vi "MultiPAS-IV.vi"() -> ()   [LabVIEW 2011]
uses:
  <vilib>/Analysis/4window.llb/windowTd.ctl
  sub/QMH/QMH Add Message to Queue (Single Element).vi
  sub/QMH/QMH Add Message to Queue (Array).vi
  sub/laserDiagnose_IV.vi
  <vilib>/Instr/_visa.llb/VISA Configure Serial Port (Instr).vi
  sub/lasersSetFrequencies_IV.vi
  sub/absCalcPlot_IV.vi
  <vilib>/measure/maspectr.llb/FFT Spectrum (Mag-Phase) for 1 Chan.vi
  sub/fftGetMags_IV.vi
  sub/rollingAverage_IV.vi
  sub/micUnbundle_IV.vi
  sub/pdNormalize_IV.vi
  <vilib>/measure/NI_MAPro.lvlib
  <vilib>/Analysis/NI_AALPro.lvlib
panel:
  in  "785 Emission":bool
  in  "785 Power (mW)":dbl(slide)=100.0 min=0.0 max=100.0 step=1.0 scale=0.0..100.0
  out "PAS Save":bool caption="Overtemp"
  in  "Data 2":i32[][](array[numeric])=[[-16374, -7248, 2543, 12030, 20279, 26487, 30037, 30583, 28073, 22744, 15131, 5976, -3818, -13288, -21504, -27663, -31155, -31636, -29064, -23686, -16036, -6862, 2936, 12388, 20571, 26684, 30122, 30546, 27911, 22483, 14793, 5595, -4207, -13644, -21795, -27855, -31232, -31591, -28898, -23423, -15695, -6476, 3323, 12743, 20858, 26873, 30194, 30492, 27744, 22213, 14447, 5207, -4597, -14002, -22082, -28044, -31304, -31540, -28731, -23149, -15348, -6093, 3713, 13101, 21145, 27063, 30265, 30442, 27576, 21943, 14103, 4822, -4984, -14354, -22365, -28230, -31373, -31485, -28556, -22876, -14998, -5702, 4104, 13452, 21428, 27245, 30335, 30388, 27400, 21669, 13754, 4435, -5375, -14705, -22643, -28407, -31436, -31426, -28378, -22598, -14648, -5314, 4497, 13803, 21706, 27423, 30394, 30325, 27221, 21390, 13402, 4045, -5763, -15056, -22921, -28586, -31496, -31361, -28198, -22319, -14297, -4924, 4879, 14151, 21982, 27597, 30451, 30257, 27038, 21107, 13050, 3658, -6149, -15402, -23193, -28754, -31546, -31290, -28010, -22033, -13944, -4536, 5266, 14498, 22252, 27767, 30500, 30184, 26849, 20821, 12696, 3267, -6535, -15748, -23462, -28924, -31596, -31216, -27821, -21748, -13587, -4147, 5653, 14838, 22519, 27930, 30549, 30110, 26658, 20535, 12337, 2878, -6919, -16089, -23727, -29087, -31641, -31137, -27627, -21457, -13229, -3753, 6038, 15181, 22786, 28093, 30591, 30031, 26461, 20243, 11979, 2485, -7303, -16428, -23991, -29244, -31678, -31053, -27426, -21159, -12867, -3360, 6424, 15524, 23043, 28252, 30633, 29946, 26262, 19946, 11617, 2096, -7686, -16764, -24246, -29398, -31712, -30964, -27224, -20862, -12503, -2971, 6803, 15859, 23301, 28401, 30661, 29852, 26058, 19648, 11254, 1703, -8069, -17099, -24500, -29547, -31741, -30870, -27018, -20562, -12138, -2575, 7188, 16192, 23556, 28549, 30689, 29756, 25848, 19348, 10891, 1312, -8448, -17430, -24753, -29691, -31765, -30773, -26806, -20259, -11775, -2186, 7566, 16521, 23801, 28690, 30709, 29656, 25634, 19038, 10523, 919, -8831, -17762, -24997, -29833, -31788, -30672, -26593, -19955, -11409, -1792, 7944, 16850, 24047, 28830, 30724, 29548, 25416, 18729, 10152, 523, -9212, -18092, -25245, -29969, -31805, -30566, -26375, -19647, -11041, -1403, 8319, 17173, 24287, 28963, 30734, 29436, 25192, 18418, 9781, 130, -9587, -18413, -25481, -30101, -31814, -30449, -26150, -19332, -10666, -1007, 8697, 17497, 24524, 29090, 30745, 29325, 24968, 18105, 9408, -263, -9962, -18735, -25718, -30228, -31820, -30334, -25921, -19016, -10296, -618, 9072, 17814, 24756, 29213, 30746, 29202, 24738, 17787, 9036, -657, -10338, -19058, -25951, -30350, -31818, -30214, -25690, -18699, -9922, -224, 9442, 18128, 24984, 29330, 30738, 29078, 24502, 17466, 8658, -1050, -10710, -19371, -26178, -30467, -31814, -30088, -25458, -18382, -9550, 167, 9812, 18440, 25206, 29443, 30732, 28947, 24264, 17143, 8281, -1445, -11083, -19685, -26404, -30581, -31807, -29959, -25221, -18059, -9175, 556, 10178, 18750, 25426, 29548, 30718, 28809, 24018, 16812, 7901, -1842, -11457, -19996, -26624, -30690, -31795, -29824, -24980, -17733, -8799, 950, 10549, 19058, 25643, 29655, 30700, 28673, 23773, 16484, 7523, -2235, -11824, -20304, -26840, -30793, -31772, -29682, -24731, -17402, -8415, 1341, 10916, 19363, 25856, 29755, 30677, 28528, 23522, 16151, 7141, -2626, -12191, -20607, -27051, -30891, -31746, -29536, -24481, -17070, -8035, 1733, 11280, 19664, 26064, 29851, 30648, 28381, 23272, 15818, 6762, -3019, -12555, -20906, -27258, -30984, -31717, -29391, -24226, -16736, -7655, 2128, 11641, 19962, 26270, 29940, 30615, 28229, 23013, 15483, 6376, -3409, -12914, -21204, -27459, -31071, -31684, -29236, -23967, -16398, -7271, 2515, 12005, 20258, 26468, 30024, 30577, 28072, 22753, 15143, 5990, -3802, -13276, -21497, -27660, -31157, -31643, -29076, -23707, -16058, -6886, 2908, 12363, 20550, 26666, 30107, 30536, 27914, 22489, 14805, 5607, -4192, -13633, -21787, -27849, -31230, -31597, -28911, -23438, -15716, -6501, 3298, 12719, 20839, 26858, 30182, 30488, 27744, 22223, 14459, 5225, -4579, -13988, -22071, -28040, -31304, -31549, -28743, -23167, -15368, -6113, 3693, 13076, 21126, 27047, 30255, 30438, 27576, 21950, 14113, 4837, -4971, -14340, -22354, -28224, -31375, -31494, -28570, -22895, -15022, -5725, 4080, 13430, 21408, 27230, 30324, 30384, 27402, 21676, 13766, 4449, -5360, -14694, -22636, -28409, -31440, -31436, -28397, -22617, -14674, -5338, 4467, 13781, 21686, 27408, 30385, 30320, 27224, 21398, 13418, 4062, -5748, -15044, -22913, -28584, -31498, -31368, -28212, -22339, -14321, -4948, 4856, 14131, 21963, 27583, 30440, 30254, 27042, 21118, 13062, 3669, -6137, -15390, -23183, -28751, -31551, -31297, -28024, -22049, -13962, -4556, 5245, 14476, 22235, 27754, 30497, 30186, 26857, 20834, 12710, 3283, -6519, -15733, -23453, -28921, -31600, -31226, -27837, -21765, -13610, -4168, 5628, 14820, 22502, 27918, 30540, 30109, 26664, 20544, 12354, 2891, -6906, -16074, -23719, -29085, -31646, -31148, -27642, -21475, -13251, -3777, 6014, 15160, 22765, 28078, 30583, 30027, 26468, 20251, 11994, 2501, -7292, -16415, -23980, -29242, -31682, -31064, -27443, -21181, -12892, -3386, 6397, 15501, 23026, 28238, 30624, 29944, 26269, 19959, 11633, 2110, -7673, -16753, -24239, -29395, -31719, -30974, -27239, -20882, -12528, -2993, 6782, 15835, 23285, 28390, 30651, 29852, 26063, 19660, 11271, 1720, -8053, -17087, -24493, -29546, -31746, -30880, -27031, -20583, -12163, -2599, 7166, 16173, 23538, 28538, 30684, 29758, 25853, 19356, 10906, 1327, -8433, -17416, -24743, -29688, -31769, -30782, -26821, -20280, -11797, -2208, 7543, 16501, 23786, 28680, 30704, 29656, 25642, 19053, 10540, 936, -8814, -17747, -24989, -29827, -31787, -30678, -26606, -19973, -11430, -1817, 7923, 16829, 24031, 28819, 30721, 29552, 25424, 18746, 10174, 543, -9191, -18072, -25231, -29962, -31802, -30567, -26384, -19660, -11057, -1422, 8302, 17159, 24274, 28952, 30738, 29443, 25205, 18435, 9801, 150, -9568, -18401, -25472, -30095, -31811, -30457, -26163, -19349, -10687, -1031, 8679, 17481, 24511, 29082, 30742, 29327, 24979, 18121, 9431, -241, -9943, -18717, -25707, -30221, -31815, -30337, -25930, -19029, -10312, -631, 9058, 17802, 24745, 29207, 30746, 29209, 24750, 17805, 9057, -634, -10316, -19037, -25937, -30340, -31814, -30217, -25700, -18713, -9939, -240, 9429, 18117, 24976, 29328, 30740, 29088, 24519, 17486, 8682, -1027, -10688, -19352, -26164, -30458, -31810, -30091, -25465, -18390, -9561, 154, 9800, 18433, 25201, 29442, 30735, 28959, 24282, 17165, 8308, -1420, -11063, -19665, -26386, -30570, -31801, -29961, -25227, -18068, -9185, 547, 10171, 18745, 25424, 29552, 30726, 28825, 24038, 16835, 7925, -1815, -11429, -19974, -26608, -30681, -31789, -29826, -24984, -17741, -8807, 938, 10536, 19047, 25636, 29657, 30708, 28685, 23794, 16510, 7550, -2205, -11798, -20280, -26821, -30782, -31766, -29684, -24737, -17411, -8429, 1331, 10906, 19356, 25851, 29758, 30684, 28544, 23546, 16178, 7169, -2598, -12162, -20582, -27035, -30879, -31744, -29540, -24485, -17080, -8048, 1721, 11267, 19655, 26061, 29852, 30654, 28395, 23291, 15843, 6786, -2993, -12527, -20884, -27240, -30974, -31713, -29390, -24230, -16744, -7662, 2115, 11635, 19957, 26268, 29945, 30624, 28246, 23035, 15509, 6406, -3382, -12889, -21180, -27444, -31061, -31677, -29236, -23975, -16408, -7284], [-19329, -1252, 17344, 29341, 30145, 19451, 1353, -17227, -29174, -29920, -19175, -1056, 17506, 29408, 30095, 19300, 1159, -17387, -29238, -29860, -19019, -860, 17671, 29475, 30037, 19143, 960, -17553, -29307, -29809, -18866, -664, 17832, 29545, 29987, 18991, 771, -17707, -29365, -29749, -18707, -466, 17992, 29605, 29926, 18832, 570, -17873, -29434, -29694, -18556, -272, 18151, 29670, 29869, 18676, 375, -18031, -29495, -29633, -18395, -75, 18310, 29729, 29809, 18516, 175, -18194, -29561, -29579, -18238, 120, 18469, 29792, 29750, 18362, -17, -18347, -29617, -29515, -18076, 316, 18629, 29848, 29682, 18197, -218, -18510, -29679, -29456, -17921, 513, 18787, 29910, 29626, 18042, -408, -18664, -29734, -29388, -17757, 709, 18941, 29965, 29560, 17875, -609, -18823, -29791, -29326, -17600, 904, 19095, 30023, 29495, 17717, -802, -18975, -29845, -29260, -17434, 1099, 19251, 30075, 29425, 17551, -1001, -19131, -29901, -29194, -17277, 1296, 19408, 30130, 29359, 17393, -1193, -19284, -29953, -29124, -17112, 1491, 19560, 30184, 29290, 17225, -1392, -19440, -30008, -29056, -16949, 1686, 19713, 30237, 29226, 17069, -1581, -19587, -30054, -28982, -16781, 1883, 19866, 30287, 29151, 16898, -1781, -19742, -30107, -28913, -16616, 2079, 20018, 30337, 29082, 16737, -1973, -19888, -30152, -28838, -16449, 2275, 20167, 30383, 29006, 16564, -2174, -20041, -30200, -28765, -16282, 2471, 20321, 30430, 28934, 16403, -2364, -20187, -30243, -28688, -16113, 2669, 20465, 30470, 28853, 16230, -2568, -20341, -30294, -28618, -15953, 2860, 20615, 30519, 28783, 16070, -2755, -20486, -30335, -28537, -15779, 3057, 20760, 30560, 28700, 15892, -2956, -20637, -30378, -28461, -15613, 3252, 20909, 30605, 28628, 15730, -3145, -20777, -30418, -28377, -15440, 3446, 21054, 30645, 28543, 15557, -3345, -20927, -30460, -28299, -15271, 3643, 21199, 30686, 28465, 15391, -3534, -21066, -30495, -28215, -15100, 3839, 21345, 30722, 28380, 15214, -3734, -21213, -30534, -28134, -14928, 4032, 21487, 30760, 28300, 15044, -3926, -21355, -30570, -28052, -14757, 4225, 21627, 30792, 28209, 14870, -4123, -21501, -30607, -27968, -14586, 4419, 21768, 30832, 28129, 14702, -4314, -21637, -30639, -27880, -14413, 4612, 21907, 30859, 28040, 14521, -4515, -21780, -30675, -27796, -14241, 4804, 22048, 30895, 27953, 14352, -4702, -21919, -30705, -27707, -14064, 4999, 22187, 30922, 27859, 14172, -4900, -22060, -30739, -27620, -13892, 5193, 22326, 30954, 27773, 14003, -5090, -22194, -30765, -27524, -13712, 5386, 22462, 30981, 27679, 13823, -5285, -22333, -30794, -27436, -13538, 5580, 22600, 31013, 27591, 13650, -5476, -22466, -30820, -27343, -13363, 5770, 22732, 31033, 27491, 13468, -5673, -22605, -30848, -27251, -13187, 5964, 22870, 31060, 27401, 13292, -5863, -22736, -30870, -27155, -13010, 6156, 23000, 31079, 27299, 13111, -6058, -22873, -30895, -27060, -12833, 6347, 23134, 31104, 27208, 12936, -6248, -23004, -30918, -26965, -12652, 6536, 23260, 31120, 27106, 12753, -6444, -23136, -30939, -26865, -12472, 6729, 23395, 31148, 27011, 12578, -6634, -23266, -30959, -26766, -12296, 6919, 23523, 31161, 26907, 12392, -6830, -23402, -30982, -26665, -12115, 7109, 23652, 31180, 26809, 12213, -7016, -23524, -30992, -26564, -11932, 7301, 23777, 31195, 26704, 12032, -7210, -23655, -31011, -26464, -11755, 7492, 23907, 31211, 26605, 11855, -7395, -23778, -31024, -26358, -11573, 7680, 24031, 31218, 26494, 11665, -7592, -23908, -31039, -26258, -11392, 7871, 24158, 31237, 26394, 11491, -7775, -24031, -31050, -26153, -11210, 8063, 24281, 31247, 26285, 11302, -7972, -24159, -31062, -26046, -11027, 8250, 24407, 31258, 26180, 11124, -8157, -24276, -31067, -25937, -10841, 8438, 24526, 31265, 26071, 10936, -8347, -24401, -31078, -25829, -10659, 8630, 24649, 31275, 25965, 10755, -8533, -24522, -31087, -25721, -10474, 8816, 24770, 31280, 25853, 10566, -8726, -24641, -31091, -25608, -10290, 9003, 24891, 31287, 25746, 10386, -8910, -24756, -31095, -25498, -10105, 9192, 25008, 31287, 25627, 10196, -9102, -24881, -31101, -25386, -9919, 9381, 25127, 31296, 25521, 10019, -9284, -24994, -31099, -25268, -9732, 9570, 25243, 31293, 25403, 9826, -9476, -25113, -31105, -25157, -9544, 9756, 25359, 31298, 25291, 9645, -9655, -25225, -31099, -25040, -9359, 9942, 25473, 31291, 25167, 9453, -9847, -25341, -31102, -24926, -9173, 10124, 25586, 31294, 25057, 9269, -10029, -25450, -31095, -24809, -8986, 10310, 25696, 31284, 24931, 9078, -10218, -25564, -31094, -24688, -8798, 10497, 25812, 31287, 24819, 8896, -10399, -25673, -31085, -24567, -8608, 10682, 25922, 31278, 24698, 8703, -10587, -25785, -31080, -24448, -8422, 10866, 26033, 31274, 24582, 8522, -10765, -25890, -31067, -24321, -8230, 11050, 26140, 31263, 24455, 8325, -10952, -26001, -31064, -24201, -8040, 11234, 26248, 31255, 24338, 8142, -11132, -26106, -31054, -24079, -7852, 11417, 26353, 31243, 24207, 7948, -11316, -26217, -31041, -23952, -7662, 11601, 26464, 31236, 24089, 7763, -11494, -26315, -31025, -23829, -7471, 11782, 26562, 31217, 23957, 7567, -11682, -26422, -31014, -23702, -7282, 11962, 26667, 31205, 23834, 7383, -11859, -26521, -30998, -23575, -7092, 12144, 26770, 31187, 23704, 7186, -12043, -26626, -30981, -23444, -6900, 12328, 26875, 31176, 23582, 7003, -12218, -26724, -30962, -23316, -6709, 12505, 26971, 31154, 23446, 6805, -12401, -26825, -30946, -23189, -6517, 12687, 27073, 31139, 23322, 6620, -12576, -26919, -30922, -23054, -6323, 12867, 27170, 31114, 23185, 6422, -12760, -27022, -30904, -22923, -6132, 13047, 27272, 31096, 23060, 6237, -12934, -27114, -30879, -22790, -5940, 13222, 27362, 31068, 22921, 6041, -13116, -27212, -30855, -22657, -5748, 13401, 27461, 31048, 22790, 5853, -13289, -27302, -30828, -22522, -5555, 13577, 27549, 31019, 22652, 5652, -13472, -27398, -30806, -22388, -5362, 13753, 27645, 30995, 22521, 5463, -13642, -27487, -30776, -22248, -5169, 13928, 27733, 30963, 22376, 5266, -13823, -27584, -30750, -22113, -4975, 14106, 27828, 30937, 22246, 5082, -13992, -27669, -30717, -21974, -4782, 14280, 27914, 30902, 22101, 4880, -14174, -27760, -30689, -21837, -4588, 14454, 28006, 30875, 21965, 4692, -14340, -27843, -30653, -21693, -4391, 14631, 28092, 30840, 21822, 4494, -14519, -27934, -30620, -21552, -4198, 14805, 28179, 30808, 21688, 4308, -14687, -28015, -30582, -21410, -4004, 14975, 28262, 30770, 21540, 4106, -14861, -28103, -30548, -21268, -3808, 15149, 28349, 30739, 21402, 3916, -15032, -28183, -30512, -21124, -3614, 15319, 28430, 30697, 21255, 3715, -15205, -28267, -30475, -20982, -3421, 15490, 28513, 30664, 21116, 3524, -15376, -28348, -30435, -20837, -3225, 15660, 28592, 30617, 20962, 3327, -15550, -28432, -30397, -20695, -3032, 15829, 28673, 30581, 20820, 3134, -15711, -28506, -30353, -20546, -2837, 15994, 28746, 30530, 20669, 2933, -15887, -28585, -30311, -20400, -2641, 16167, 28828, 30496, 20528, 2745, -16052, -28660, -30264, -20248, -2445, 16335, 28901, 30445, 20376, 2544, -16221, -28737, -30219, -20102, -2250, 16505, 28983, 30406, 20231, 2357, -16381, -28808, -30171, -19950, -2053, 16670, 29053, 30355, 20075, 2154, -16552, -28883, -30127, -19803, -1859, 16835, 29128, 30308, 19930, 1965, -16714, -28952, -30073, -19650, -1663, 17001, 29192, 30255, 19772, 1764, -16881, -29028, -30026, -19496, -1467, 17165, 29268, 30208, 19626, 1572, -17043, -29095, -29977, -19346]]
  out "Filtering":bool caption="Time has Elapsed"
  in  "Switch Filter":bool
  in  "Auto Filter":bool
  out "Elapsed Time (min)":dbl caption="Elapsed Time (s)" format="%#.1g"
  in  "Filter Length (min)":dbl=6.0 caption="Time Target (s)"
  in  "Sample Length (min)":dbl=24.0 caption="Time Target (s)" format="%#.1f"
  out "Time has Elapsed":bool
  in  "Time Target (s)":dbl=1.0
  in  "sweep":bool
  in  "All Emit":bool
  in  "Alignment Mode":bool
  in  "662 Emission":bool
  in  "662 Power (mW)":dbl(slide)=100.0 min=0.0 max=100.0 step=1.0 scale=0.0..100.0
  in  "532 Emission":bool
  in  "532 Power (mW)":dbl(slide)=100.0 min=0.0 max=80.0 step=1.0 scale=0.0..80.0
  in  "406 Power (mW)":dbl(slide)=100.0 min=0.0 max=100.0 step=1.0 scale=0.0..100.0
  in  "406 Emission":bool
  out "Overtemp":bool
  in  "Tab Control":T1(tab)=enum."Frequency Sweep"
  out "crd":path
  in  "785 Port":refnum<visa-resource-name>="COM81"
  in  "785 PD Cal":dbl=0.793
  out "Error Console":T2
  out "pd":path caption="Photodiode File Path"
  out "mic":path caption="Microphone File Path"
  out "processed":path caption="Processed Data File Path"
  out "sweeps":path caption="Frequency Sweeps File Path"
  out "Laser Temperatures":T3(graph)
  in  "pd id":u32=1
  in  "mic id":u32
  in  "mic cal, scu":dbl=5.41531278804282e-05 format="%#_3e"
  in  "mic cal, scu":dbl=5.59307241877627e-05 format="%#_3e"
  in  "406 Port":refnum<visa-resource-name>="COM80"
  in  "532 Port":refnum<visa-resource-name>="COM79"
  in  "662 Port":refnum<visa-resource-name>="COM62"
  in  "Teensy Port":refnum<visa-resource-name>="COM78"
  in  "Save Data":bool
  in  "405 PD Cal 3":dbl=0.237
  in  "532 PD Cal 3":dbl=0.454
  in  "660 PD Cal 3":dbl=0.793
  in  "785 F (Hz)":i32=1370
  out "freqscan":cluster{i32[], "Best Gaussian Fit":dbl[]}[](graph) caption="Frequency Sweep"
  out "sweep progress":dbl(slide) scale=0.0..1.0
  in  "Autosweep?":bool=TRUE
  in  "set freqs":bool
  out "Calculated Resonance (Hz)":dbl=1370.0
  in  "Data Start Frequency (Hz)":i32=1355
  in  "Data End Frequency (Hz)":i32=1385
  in  "423 F (Hz)":i32=1368
  in  "532 F (Hz)":i32=1372
  in  "662 F (Hz)":i32=1370
  in  "Chart Rolling Average":i32=64
  out "pdwave":waveform(i32)(graph) caption="Photodiode Waveform"
  out "pd ts":cluster{dbl, dbl, dbl, dbl}(graph)
  out "pdfft":cluster{"f0":dbl, "df":dbl, "magnitude":dbl[]}(graph) caption="Photodiode FFT"
  in  "rollavg":i32=16 caption="Dispaly Averaging\n(Transfers to Abs!)"
  out "mic ts":T4(graph)
  out "micfft":cluster{"f0":dbl, "df":dbl, "magnitude":dbl[]}(graph) caption="Photodiode FFT"
  out "micwave":waveform(i32)(graph) caption="Photodiode Waveform"
  out "abs/ext":cluster{dbl, dbl, dbl, dbl, "crd":dbl}(graph)
  in  "getbkg":bool
  out "AAE":dbl(graph)
  in  "Bkg Values (mV)":cluster{dbl, dbl, dbl, dbl}
  out "Absorption Spectrum":cluster{dbl[], "Best Power Fit":dbl[]}[](graph)
  in  "cellcal":dbl=100000.0 caption="Cell Calibration Coefficient (mV/mW)"
  in  "fast":bool=TRUE
  out "b_ext (1/Mm)":dbl
  out "Decay":cluster{sgl[], "Best Exponential Fit":dbl[]}[](graph)
  out "Tau_662 vs. T":dbl(graph)
  in  "No. Averages":i32=96 min=1
  in  "tau_0 (us)":dbl
  out "Status":string
  in  "Exit":bool
  in  "State Variables":cluster{"CurrentFile":path}
  # "MultiPAS-IV | AeroSmith Labs (2017)"
  # "Laser Control"
  # "Filter Control"
  # "Communications"
  # "Sound Card Parameters"
  # "File paths are populated automatically at <...\\My Documents\\MultiPAS Data\\>.  To save in another location, turn on \"Save Data\" and follow the prompts to choose an alternate working directory."
  # "Photodiode Calibration"
  # "Ringdown Time (us):"
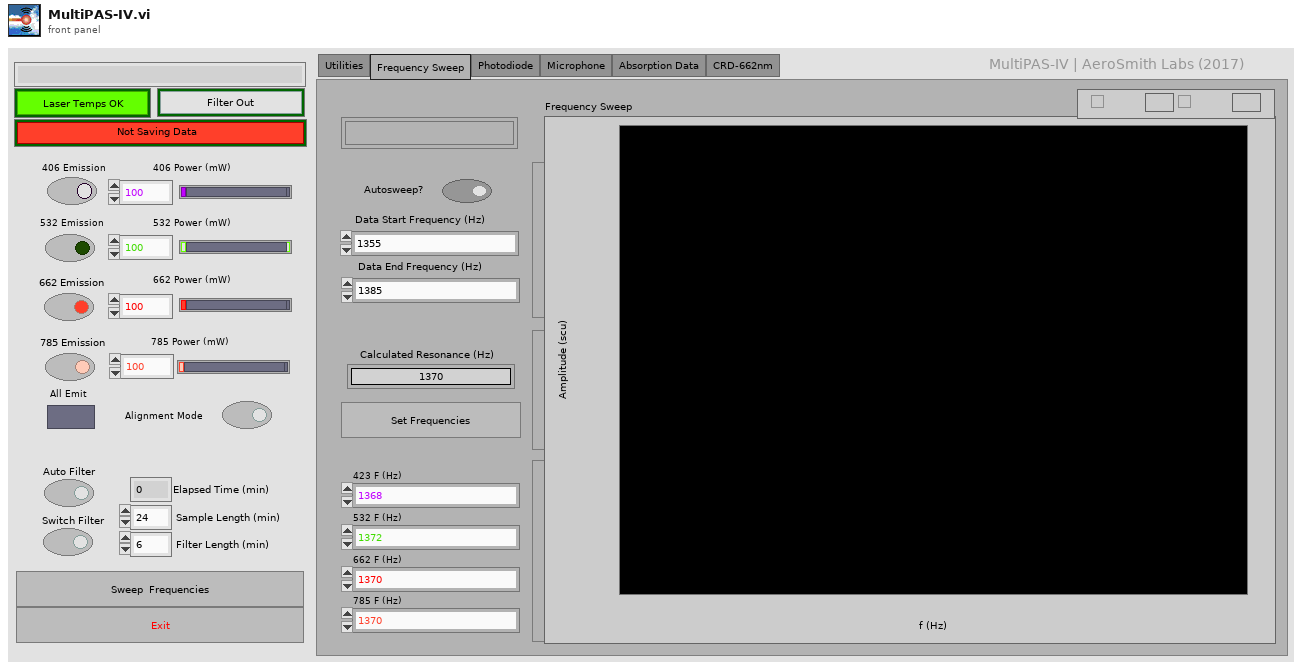
[diagram p1: front panel]
types:
  T1 = enum32{"Utilities", "Frequency Sweep", "Photodiode", "Microphone", "Absorption Data", "CRD-662nm"}
  T2 = cluster{"status":bool, "code":i32, "Message":string}
  T3 = cluster{"Temp (C)":dbl, "Temp (C)":dbl, "Temp (C)":dbl, "Temp (C)":dbl}
  T4 = cluster{"422 Mean":dbl, "532 Mean":dbl, "660 Mean":dbl, "785 Mean":dbl}
  T5 = cluster{i32, "Sample Internal":sgl, "Data (Volts)":dbl[]}
  T6 = cluster{"# buffers":i32, "Buffer size":i32, "unit (ms)":enum16{"time (ms)", "Samples"}}
  T7 = typedef "SoundHandle.ctl" = cluster{"DeviceID":u16, "Samples/buf":u32, "Sampl rate":u32, "Bits/sample":u16, "Channels":u8, "Opened":bool}
  T8 = cluster{"Driver Version":string, "USB Version":string, "Hardware":string, "Variant":string, "Batch and Serial":string, "Cal Date":string, "Kernel Version":string, "Digital HW Version":string, "Analogue HW Version":string, "Firmware 1":string, "Firmware 2":string, "MSO":bool, "Number of Channels":i16}
  T9 = cluster{"405 Mean":dbl, "532 Mean":dbl, "660 Mean":dbl, "660 Mean 2":dbl}
  T10 = typedef "NI_AALPro.lvlib/windowTd.ctl" = u32
  T11 = cluster{"785 New Array":dbl[], "785 Mean":dbl, "785 SD":dbl}
  T12 = cluster{"660 New Array":dbl[], "660 Mean":dbl, "660 SD":dbl}
  T13 = cluster{"532 New Array":dbl[], "532 Mean":dbl, "532 SD":dbl}
  T14 = cluster{"405 New Array":dbl[], "405 Mean":dbl, "405 SD":dbl}
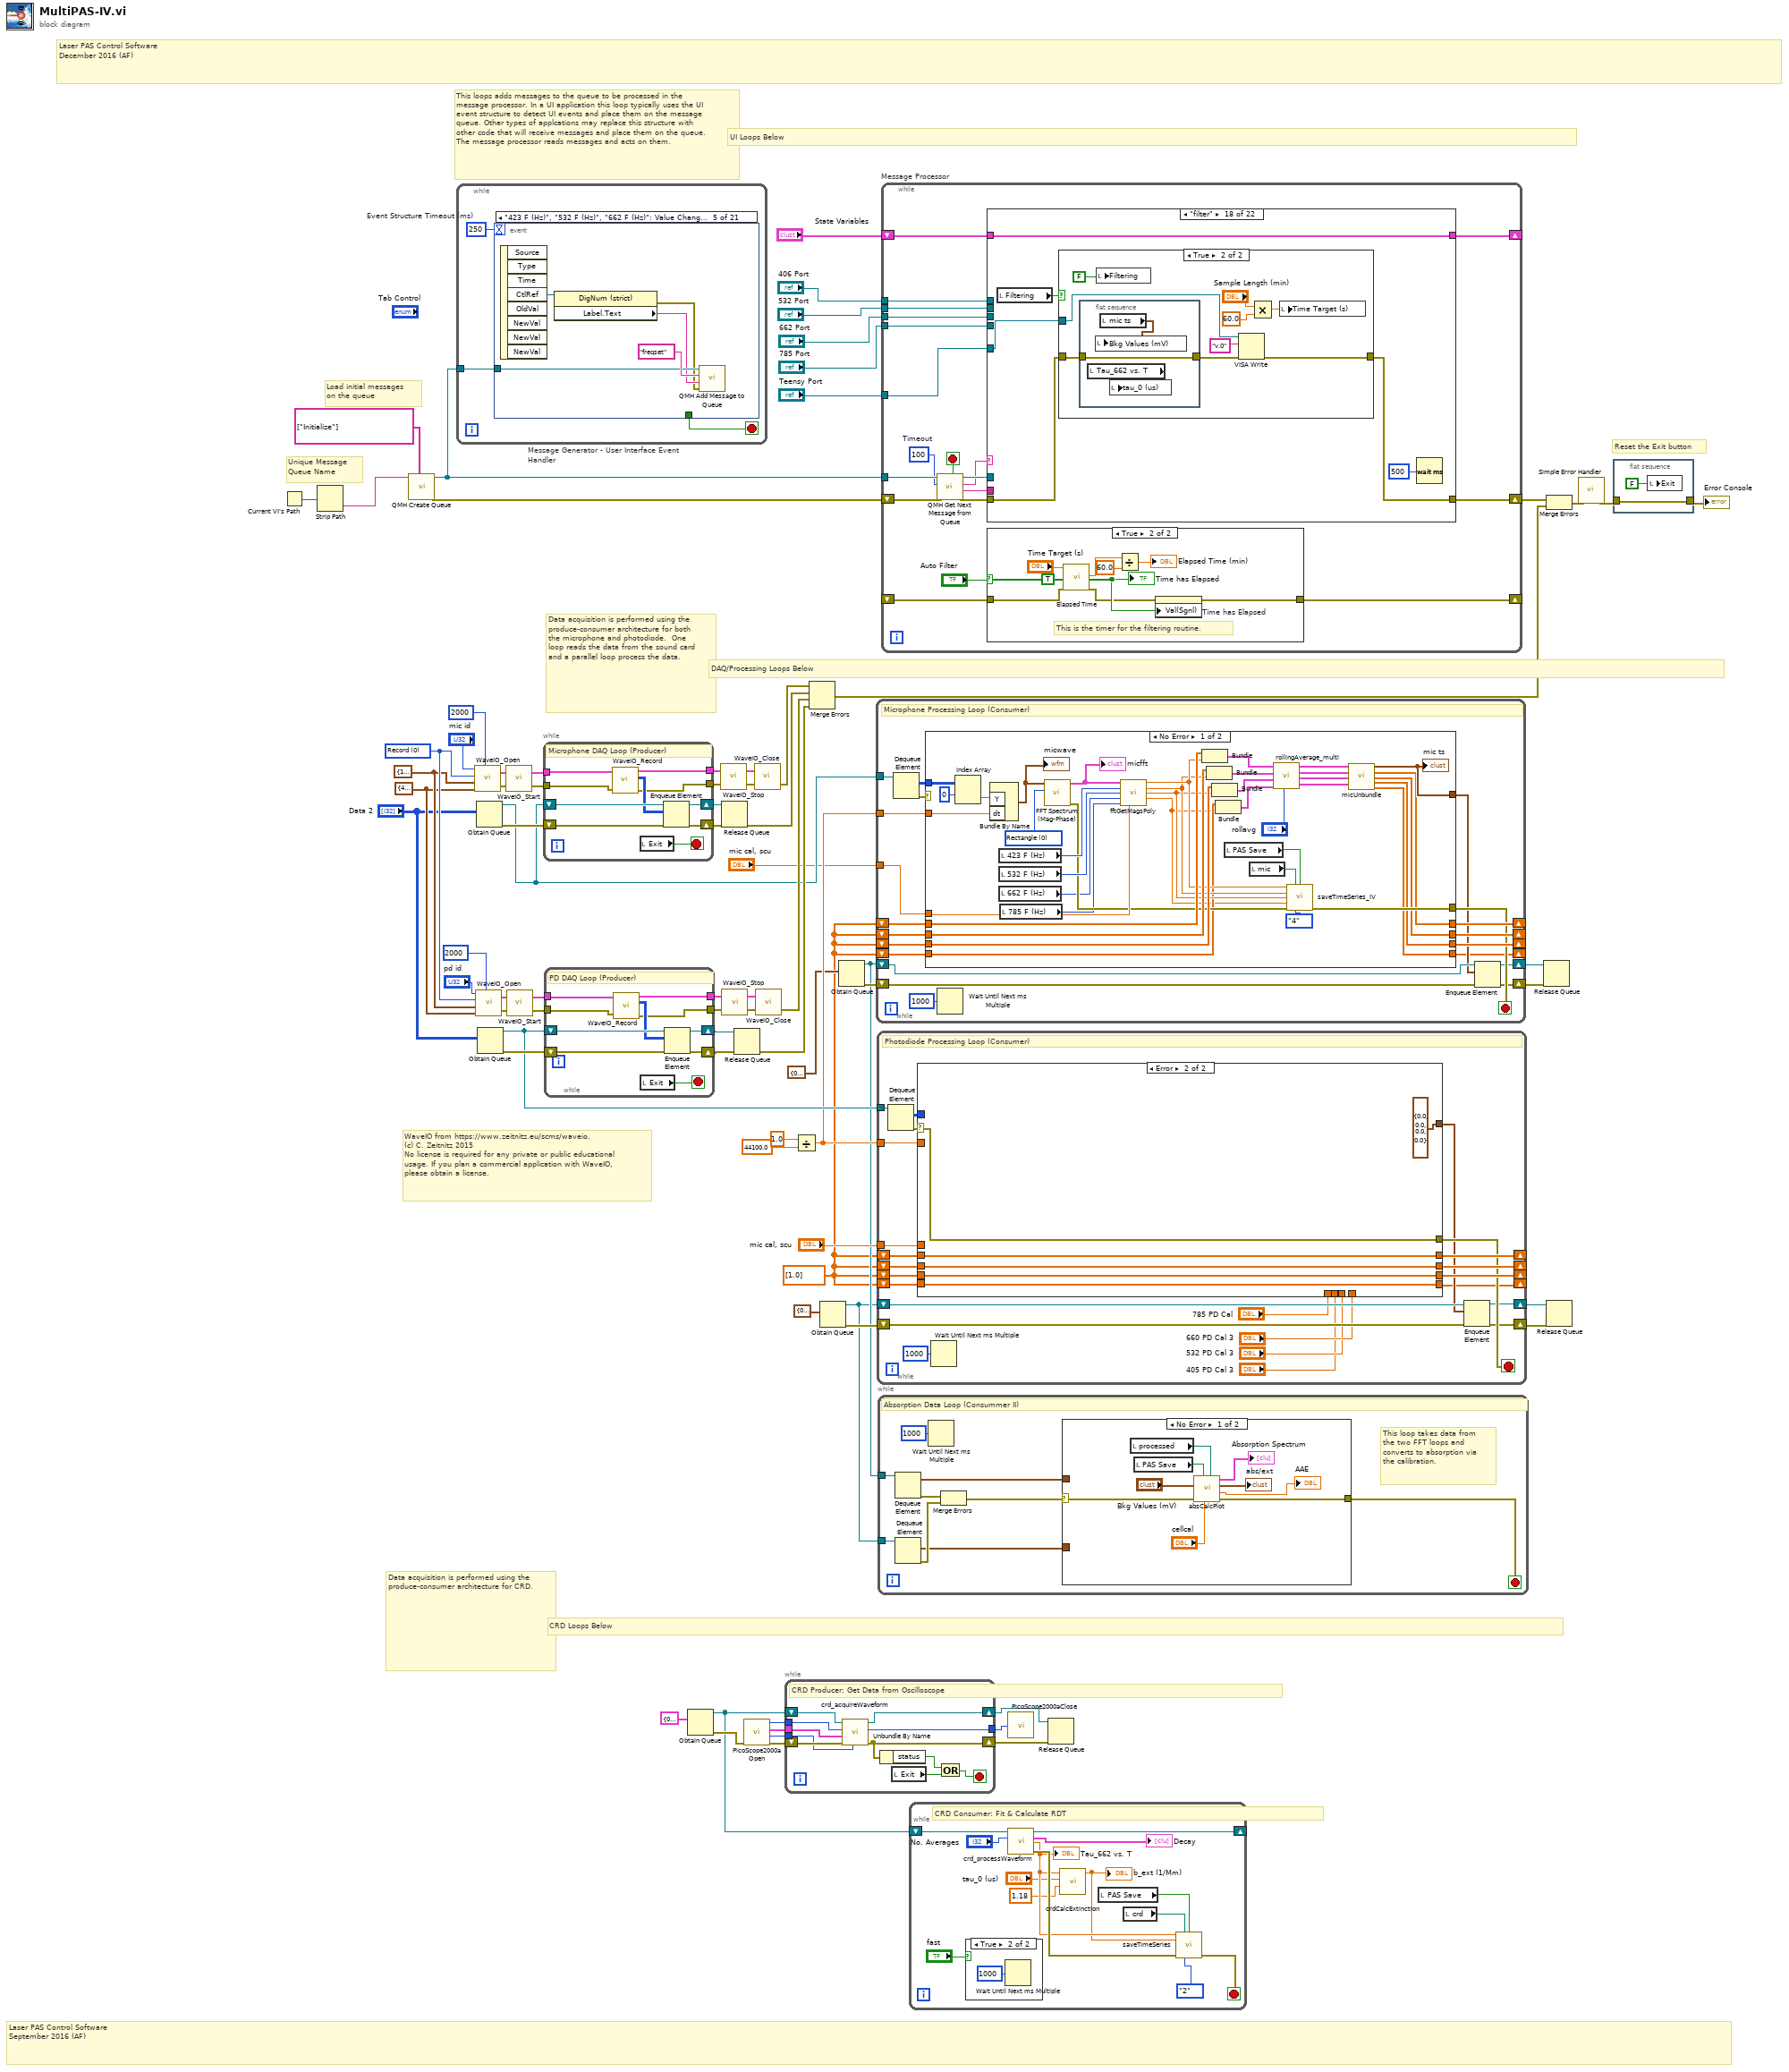
[diagram p0: block diagram]
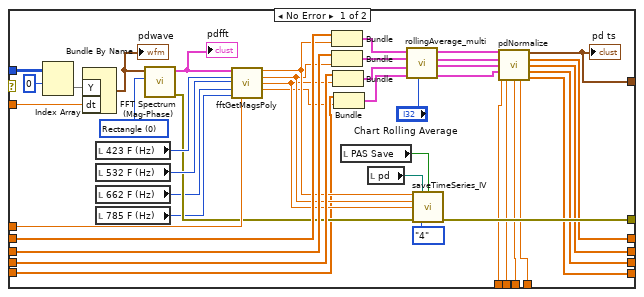
[diagram p4: hidden frame]
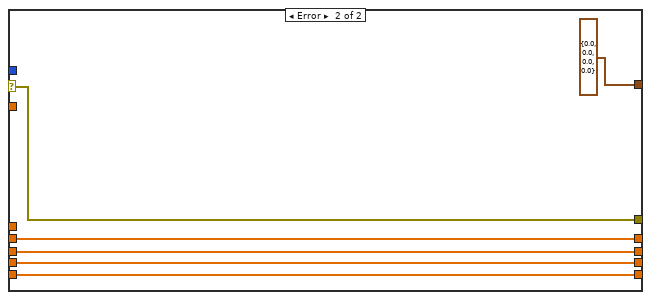
[diagram p5: hidden frame]
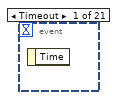
[diagram p6: hidden frame]
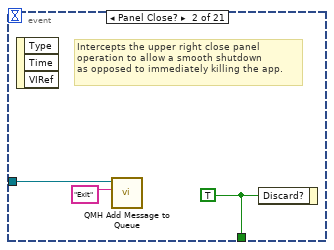
[diagram p7: hidden frame]
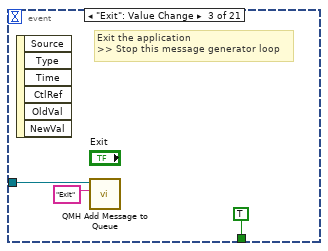
[diagram p8: hidden frame]
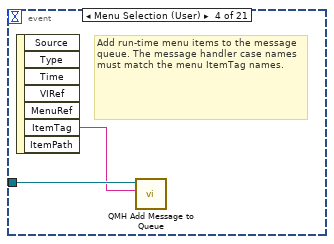
[diagram p9: hidden frame]
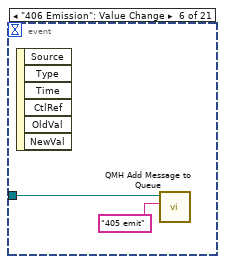
[diagram p10: hidden frame]
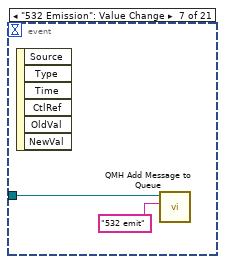
[diagram p11: hidden frame]
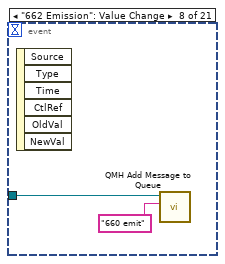
[diagram p12: hidden frame]
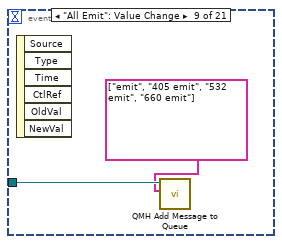
[diagram p13: hidden frame]
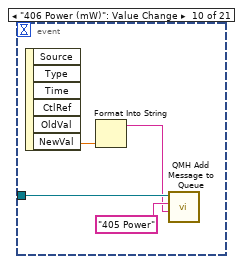
[diagram p14: hidden frame]
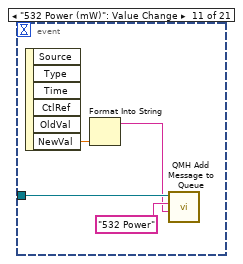
[diagram p15: hidden frame]
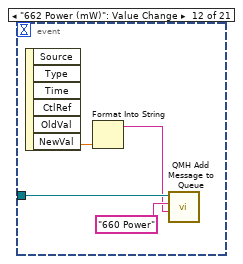
[diagram p16: hidden frame]
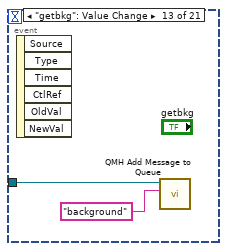
[diagram p17: hidden frame]
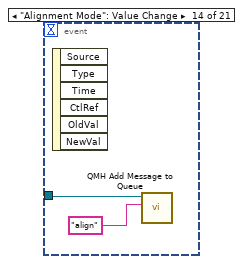
[diagram p18: hidden frame]
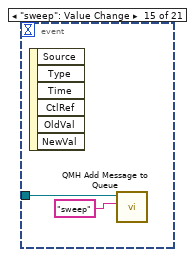
[diagram p19: hidden frame]
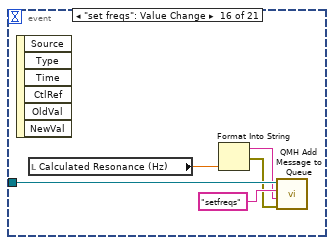
[diagram p20: hidden frame]
diagram:
  w32 = T6 {"# buffers"=10, "Buffer size"=44100, "unit (ms)"=enum."Samples"} ("Buffer")
  w31 = cluster{"Rate":i32, "Bits":i32, "Channels":i32} {"Rate"=44100, "Bits"=24, "Channels"=2} ("Format")
  w33 = u16 0 items=["Record", "Play", "Loopback", "ASIO input", "ASIO output"] ("Direction (Record)")
  w12 = dbl[] [1.0] ("X")
  # "Data acquisition is performed using the produce-consumer architecture for CRD."
  # "CRD Loops Below"
  # "Laser PAS Control Software\nSeptember 2016 (AF)"
  # "Laser PAS Control Software\nDecember 2016 (AF)"
  # "Data acquisition is performed using the produce-consumer architecture for both the microphone and photodiode.  One loop reads the data from the sound card and a parallel loop process the data."
  # "WaveIO from https://www.zeitnitz.eu/scms/waveio.\n(c) C. Zeitnitz 2015\nNo license is required for any private or public educational usage. If you plan a commercial application with WaveIO, please obtain a license."
  # "This loops adds messages to the queue to be processed in the message processor. In a UI application this loop typically uses the UI event structure to detect UI events and place them on the message queue. Other types of applcations may replace this structure with other code that will receive messages and place them on the queue.  The message processor reads messages and acts on them."
  # "Reset the Exit button"
  # "Unique Message\nQueue Name"
  # "Load initial messages\non the queue"
  # "DAQ/Processing Loops Below"
  # "UI Loops Below"
  n1 = Current VI's Path() -> (path=w77:path)
  n2 = Strip Path(path=w77) -> (name=w78:string)  [unwired: 1 out]
  n3 = call "QMH Create Queue.vi"("Initial Messages"=string[] ["Initialize"], "Message queue name (unnamed)"=w78) -> ("error out"=w74:errorcluster, "queue out"=w60:refnum<queue>)  [unwired: 8 in]
  n4 = while "Message Generator - User Interface Event Handler" {
    tunnel: w60 -> [w79]
    stop <- w80 stop-if-true
    w81 = 250  # Event Structure Timeout (ms)
    n5 = event shown="[4] \"423 F (Hz)\", \"532 F (Hz)\", \"662 F (Hz)\": Value Change" {
      selector: _ -> [_ _ _ _ _ _ _ _ _ _ _ _ _ _ _ _ _ _ _ _ _]
      dyn-events: _ -> [_ _ _ _ _ _ _ _ _ _ _ _ _ _ _ _ _ _ _ _ _]
      timeout: w81 -> [_ _ _ _ _ _ _ _ _ _ _ _ _ _ _ _ _ _ _ _ _]
      tunnel: [_ w84 TRUE ("Discard?") _ _ _ _ _ _ _ _ _ _ _ _ _ _ _ _ _ _] -> w80
      tunnel: w79 -> [_ w83 w86 w89 w93 w95 w97 w99 w102 w105 w109 w113 w115 w117 w120 w124 w129 w134 w138 w143 w145]
      event Timeout {
        n6 = event-data() -> ()  [unwired: 1 in, 1 out]
      }
      event Panel Close? {
        w84 = TRUE ("Discard?")
        # "Intercepts the upper right close panel\noperation to allow a smooth shutdown\nas opposed to immediately killing the app."
        n7 = event-data() -> ()  [unwired: 1 in, 3 out]
        n8 = call-poly "QMH Add Message to Queue.vi"("Message"="Exit", "queue in"=w83) -> ()  [unwired: 8 in, 2 out]
        n9 = event-data("Discard?"=w84) -> ()  [unwired: 1 in, 1 out]
      }
      event "Exit": Value Change {
        # "Exit the application\n>> Stop this message generator loop"
        n10 = event-data() -> ()  [unwired: 1 in, 6 out]
        n11 = call-poly "QMH Add Message to Queue.vi"("Message"="Exit", "queue in"=w86) -> ()  [unwired: 8 in, 2 out]
      }
      event Menu Selection (User) {
        # "Add run-time menu items to the message\nqueue. The message handler case names must match the menu ItemTag names."
        n12 = event-data() -> ("ItemTag"=w88:string)  [unwired: 1 in, 6 out]
        n13 = call-poly "QMH Add Message to Queue.vi"("Message"=w88, "queue in"=w89) -> ()  [unwired: 8 in, 2 out]
      }
      event "423 F (Hz)", "532 F (Hz)", "662 F (Hz)": Value Change {
        n14 = event-data() -> ("CtlRef"=w92:refnum<vi>)  [unwired: 1 in, 7 out]
        n15 = property class="DigNum (strict)"(reference=w92) -> (error out=w90:errorcluster, "Label.Text"=w91:string)  [unwired: 1 in, 1 out]
        n16 = call-poly "QMH Add Message to Queue.vi"("error in (no error)"=w90, "Parameter"=w91, "Message"="freqset", "queue in"=w93) -> ()  [unwired: 6 in, 2 out]
      }
      event "406 Emission": Value Change {
        n17 = event-data() -> ()  [unwired: 1 in, 6 out]
        n18 = call-poly "QMH Add Message to Queue.vi"("Message"="405 emit", "queue in"=w95) -> ()  [unwired: 8 in, 2 out]
      }
      event "532 Emission": Value Change {
        n19 = event-data() -> ()  [unwired: 1 in, 6 out]
        n20 = call-poly "QMH Add Message to Queue.vi"("Message"="532 emit", "queue in"=w97) -> ()  [unwired: 8 in, 2 out]
      }
      event "662 Emission": Value Change {
        n21 = event-data() -> ()  [unwired: 1 in, 6 out]
        n22 = call-poly "QMH Add Message to Queue.vi"("Message"="660 emit", "queue in"=w99) -> ()  [unwired: 8 in, 2 out]
      }
      event "All Emit": Value Change {
        n23 = event-data() -> ()  [unwired: 1 in, 6 out]
        n24 = call-poly "QMH Add Message to Queue.vi"("Messages"=string[] ["emit", "405 emit", "532 emit", "660 emit"], "queue in"=w102) -> ()  [unwired: 8 in, 2 out]
      }
      event "406 Power (mW)": Value Change {
        n25 = event-data() -> ("NewVal"=w104:dbl)  [unwired: 1 in, 5 out]
        n26 = Format Into String(w104) -> (resulting string=w103:string)  [unwired: 3 in, 1 out]
        n27 = call-poly "QMH Add Message to Queue.vi"("Parameter"=w103, "Message"="405 Power", "queue in"=w105) -> ()  [unwired: 7 in, 2 out]
      }
      event "532 Power (mW)": Value Change {
        n28 = event-data() -> ("NewVal"=w108:dbl)  [unwired: 1 in, 5 out]
        n29 = Format Into String(w108) -> (resulting string=w107:string)  [unwired: 3 in, 1 out]
        n30 = call-poly "QMH Add Message to Queue.vi"("Parameter"=w107, "Message"="532 Power", "queue in"=w109) -> ()  [unwired: 7 in, 2 out]
      }
      event "662 Power (mW)": Value Change {
        n31 = event-data() -> ("NewVal"=w112:dbl)  [unwired: 1 in, 5 out]
        n32 = Format Into String(w112) -> (resulting string=w111:string)  [unwired: 3 in, 1 out]
        n33 = call-poly "QMH Add Message to Queue.vi"("Parameter"=w111, "Message"="660 Power", "queue in"=w113) -> ()  [unwired: 7 in, 2 out]
      }
      event "getbkg": Value Change {
        n34 = event-data() -> ()  [unwired: 1 in, 6 out]
        n35 = call-poly "QMH Add Message to Queue.vi"("Message"="background", "queue in"=w115) -> ()  [unwired: 8 in, 2 out]
      }
      event "Alignment Mode": Value Change {
        n36 = event-data() -> ()  [unwired: 1 in, 6 out]
        n37 = call-poly "QMH Add Message to Queue.vi"("Message"="align", "queue in"=w117) -> ()  [unwired: 8 in, 2 out]
      }
      event "sweep": Value Change {
        n38 = event-data() -> ()  [unwired: 1 in, 6 out]
        n39 = call-poly "QMH Add Message to Queue.vi"("Message"="sweep", "queue in"=w120) -> ()  [unwired: 8 in, 2 out]
      }
      event "set freqs": Value Change {
        n40 = event-data() -> ()  [unwired: 1 in, 6 out]
        n41 = local read "Calculated Resonance (Hz)"() -> (w123:dbl)
        n42 = Format Into String(w123) -> (resulting string=w122:string, error out=w121:errorcluster)  [unwired: 3 in]
        n43 = call-poly "QMH Add Message to Queue.vi"("error in (no error)"=w121, "Parameter"=w122, "Message"="setfreqs", "queue in"=w124) -> ()  [unwired: 6 in, 2 out]
      }
      event "Save Data": Value Change {
        n44 = event-data() -> ("NewVal"=w128:bool)  [unwired: 1 in, 5 out]
        n45 = Format Into String(w128) -> (resulting string=w127:string, error out=w126:errorcluster)  [unwired: 3 in]
        n46 = call-poly "QMH Add Message to Queue.vi"("error in (no error)"=w126, "Parameter"=w127, "Message"="namefiles", "queue in"=w129) -> ()  [unwired: 6 in, 2 out]
      }
      event "Switch Filter": Value Change {
        n47 = event-data() -> ("NewVal"=w133:bool)  [unwired: 1 in, 5 out]
        n48 = local write "Filtering"(w133) -> ()
        n49 = Format Into String(w133) -> (resulting string=w131:string)  [unwired: 3 in, 1 out]
        n50 = call-poly "QMH Add Message to Queue.vi"("Parameter"=w131, "Message"="filterswitch", "queue in"=w134) -> ()  [unwired: 7 in, 2 out]
      }
      event "Time has Elapsed": Value Change {
        n51 = event-data() -> ("NewVal"=w137:bool)  [unwired: 1 in, 5 out]
        n52 = local read "Filtering"() -> (w136:bool)
        n53 = call "filterCreateMsg.vi"("time elapsed?"=w137, "auto sweep (true)"="Autosweep?", "filtering (true)"=w136, "queue in"=w138) -> ()  [unwired: 6 in, 2 out]
      }
      event "Calculated Resonance (Hz)": Value Change {
        n54 = event-data() -> ("NewVal"=w141:dbl)  [unwired: 1 in, 5 out]
        n55 = Format Into String(w141) -> (resulting string=w139:string, error out=w140:errorcluster)  [unwired: 3 in]
        n56 = call-poly "QMH Add Message to Queue.vi"("error in (no error)"=w140, "Parameter"=w139, "Message"="setfreqs", "queue in"=w143) -> ()  [unwired: 6 in, 2 out]
      }
      event "PAS Save": Value Change {
        n57 = event-data() -> ()  [unwired: 1 in, 6 out]
        n58 = call-poly "QMH Add Message to Queue.vi"("Message"="setwd", "queue in"=w145) -> ()  [unwired: 8 in, 2 out]
      }
    }
  }
  n59 = call <userlib>:"WaveIO_Open.vi"("Watchdog timeout (msec) (default=OFF)"=2000, "Format (44kHz, 16Bit, stereo)"=w31, "Buffer Config"=w32, "Direction (Record)"=w33, "idev"="mic id") -> ("error out"=w56:errorcluster, "Sound Handle Out"=w57:T7)  [unwired: 1 in]
  n60 = call <userlib>:"WaveIO_Open.vi"("Watchdog timeout (msec) (default=OFF)"=2000, "Format (44kHz, 16Bit, stereo)"=w31, "Buffer Config"=w32, "Direction (Record)"=w33, "idev"="pd id") -> ("error out"=w42:errorcluster, "Sound Handle Out"=w41:T7)  [unwired: 1 in]
  n61 = Obtain Queue(element data type="Data 2") -> (queue out=w25:refnum<queue>, error out=w63:errorcluster)  [unwired: 4 in, 1 out]
  n62 = Obtain Queue(element data type="Data 2") -> (queue out=w29:refnum<queue>, error out=w38:errorcluster)  [unwired: 4 in, 1 out]
  n63 = call <userlib>:"WaveIO_Start.vi"("error in (no error)"=w56, "Handle"=w57) -> ("error out"=w54:errorcluster, "Handle Out"=w55:T7)
  n64 = call <userlib>:"WaveIO_Start.vi"("error in (no error)"=w42, "Handle"=w41) -> ("error out"=w44:errorcluster, "Handle Out"=w43:T7)
  n65 = while {
    shift-right: [w154] -> w64
    shift-left: w25 -> [w152]
    shift-right: [w155] -> w65
    shift-left: w63 -> [w153]
    tunnel: w55 -> [w150]
    tunnel: w54 -> [w149]
    tunnel: [w147] -> w51
    tunnel: [w146] -> w50
    stop <- w151 stop-if-true
    # "Microphone DAQ Loop (Producer)"
    n66 = call <userlib>:"WaveIO_Record.vi"("Handle"=w150, "error in (no error)"=w149) -> ("Handle Out"=w147:T7, "Data"=w148:i32[][], "error out"=w146:errorcluster)  [unwired: 1 in, 2 out]
    n67 = local read "Exit"() -> (w151:bool)
    n68 = Enqueue Element(queue=w152, element=w148, error in (no error)=w153) -> (queue out=w154:refnum<queue>, error out=w155:errorcluster)  [unwired: 1 in, 1 out]
  }
  n69 = while {
    shift-right: [w164] -> w37
    shift-left: w29 -> [w162]
    shift-right: [w165] -> w36
    shift-left: w38 -> [w163]
    tunnel: w43 -> [w160]
    tunnel: w44 -> [w159]
    tunnel: [w157] -> w47
    tunnel: [w156] -> w48
    stop <- w161 stop-if-true
    # "PD DAQ Loop (Producer)"
    n70 = call <userlib>:"WaveIO_Record.vi"("Handle"=w160, "error in (no error)"=w159) -> ("Handle Out"=w157:T7, "Data"=w158:i32[][], "error out"=w156:errorcluster)  [unwired: 1 in, 2 out]
    n71 = local read "Exit"() -> (w161:bool)
    n72 = Enqueue Element(queue=w162, element=w158, error in (no error)=w163) -> (queue out=w164:refnum<queue>, error out=w165:errorcluster)  [unwired: 1 in, 1 out]
  }
  n73 = Obtain Queue(element data type=T5 {0, "Sample Internal"=8e-09, "Data (Volts)"=array[20000 elements]} ("Channel A 2")) -> (queue out=w2:refnum<queue>, error out=w5:errorcluster)  [unwired: 4 in, 1 out]
  n74 = call <userlib>:"WaveIO_Stop.vi"("error in (no error)"=w50, "Handle"=w51) -> ("error out"=w52:errorcluster, "Handle Out"=w53:T7)
  n75 = Release Queue(queue=w64, error in (no error)=w65) -> (error out=w62:errorcluster)  [unwired: 1 in, 2 out]
  n76 = call <userlib>:"WaveIO_Stop.vi"("error in (no error)"=w48, "Handle"=w47) -> ("error out"=w46:errorcluster, "Handle Out"=w45:T7)
  n77 = Release Queue(queue=w37, error in (no error)=w36) -> (error out=w35:errorcluster)  [unwired: 1 in, 2 out]
  n78 = call "PicoScope2000aOpen.vi"("error in (no error)"=w5) -> ("error out"=w9:errorcluster, "Max Adc value"=w10:i16, "Device Info"=w8:T8, "handle"=w7:i16)  [unwired: 7 in]
  n79 = call <userlib>:"WaveIO_Close.vi"("error in (no error)"=w52, "Handle"=w53) -> ("error out"=w49:errorcluster)  [unwired: 1 out]
  n80 = call <userlib>:"WaveIO_Close.vi"("error in (no error)"=w46, "Handle"=w45) -> ("error out"=w34:errorcluster)  [unwired: 1 out]
  n81 = while {
    tunnel: w8 -> [w173]
    tunnel: w7 -> [w174]
    tunnel: w10 -> [w168]
    tunnel: [w171] -> w1
    shift-right: [w170] -> w4
    shift-left: w2 -> [w169]
    shift-right: [w167] -> w3
    shift-left: w9 -> [w175]
    stop <- w176 stop-if-true
    # "CRD Producer: Get Data from Oscilloscope"
    n82 = call "crd_acquireWaveform.vi"("Max Adc value"=w168, "error in (no error)"=w175, "Device Info"=w173, "handle"=w174, "Queue in"=w169) -> ("error out"=w167:errorcluster, "handle out"=w171:i16, "Queue out"=w170:refnum<queue>)  [unwired: 4 in]
    n83 = Unbundle By Name(w167) -> ("status"=w172:bool)
    n84 = local read "Exit"() -> (w166:bool)
    n85 = Or(x=w172, y=w166) -> (x .or. y?=w176:bool)
  }
  n86 = Divide(x=1.0, y=44100.0) -> (x/y=w26:dbl)
  n87 = Merge Errors(w49, w62, w34, w35) -> (w61:errorcluster)
  n88 = Obtain Queue(element data type=cluster{dbl, dbl, dbl, dbl} {0.0, 0.0, 0.0, 0.0}) -> (queue out=w15:refnum<queue>, error out=w19:errorcluster)  [unwired: 4 in, 1 out]
  n89 = Obtain Queue(element data type=cluster{dbl, dbl, dbl, dbl} {0.0, 0.0, 0.0, 0.0}) -> (queue out=w16:refnum<queue>, error out=w22:errorcluster)  [unwired: 4 in, 1 out]
  n90 = while {
    tunnel: w25 -> [w196]
    shift-right: [w193] -> _
    shift-left: w12 -> [w190]
    shift-right: [w192] -> _
    shift-left: w12 -> [w189]
    shift-right: [w191] -> _
    shift-left: w12 -> [w188]
    tunnel: w26 -> [w186]
    tunnel: "mic cal, scu" -> [w185]
    shift-right: [w183] -> w21
    shift-left: w16 -> [w182]
    shift-right: [w180] -> w20
    shift-left: w22 -> [w184]
    shift-right: [w178] -> _
    shift-left: w12 -> [w179]
    stop <- w187 stop-if-true
    # "Microphone Processing Loop (Consumer)"
    n91 = Dequeue Element(queue=w196) -> (element=w194:i32[][], error out=w195:errorcluster)  [unwired: 2 in, 2 out]
    n92 = case shown="No Error" w195 {
      selector: w195 -> [_ w238]
      tunnel: w194 -> [w230 _]
      tunnel: w190 -> [w234 w241]
      tunnel: w189 -> [w233 w239]
      tunnel: w188 -> [w232 w240]
      tunnel: [w207 w241] -> w193
      tunnel: [w206 w239] -> w192
      tunnel: [w205 w240] -> w191
      tunnel: [w214 w238] -> w187
      tunnel: w186 -> [w228 _]
      tunnel: w185 -> [w223 _]
      tunnel: [w208 T9 {"405 Mean"=0.0, "532 Mean"=0.0, "660 Mean"=0.0, "660 Mean 2"=0.0}] -> w181
      tunnel: w179 -> [w200 w236]
      tunnel: [w197 w236] -> w178
      frame No Error {
        w235 = T10 0 items=["Rectangle"=0, "Hanning"=1, "Hamming"=2, "Blackman-Harris"=3, "Exact Blackman"=4, "Blackman"=5, "Flat Top"=6, "4 Term B-Harris "=7, "7 Term B-Harris"=8, "Low Sidelobe"=9, "Blackman Nuttall"=11, "Triangle"=30, "Bartlett-Hanning"=31, "Bohman"=32, "Parzen"=33, "Welch"=34, "Kaiser"=60, "Dolph-Chebyshev"=61, "Gaussian"=62] ("window")
        n93 = Index Array(array=w230, index (row)=0) -> (element=w229:i32[])  [unwired: 1 in]
        n94 = Bundle By Name("Y"=w229, "dt"=w228) -> (w227:waveform(i32))  [unwired: 1 in]
        "micwave" <- w227
        n95 = local read "423 F (Hz)"() -> (w225:i32)
        n96 = local read "532 F (Hz)"() -> (w224:i32)
        n97 = local read "662 F (Hz)"() -> (w198:i32)
        n98 = local read "785 F (Hz)"() -> (w203:i32)
        n99 = call-poly <vilib>:"FFT Spectrum (Mag-Phase).vi"("window"=w235, "time signal"=w227) -> ("error out"=w215:errorcluster, "magnitude"=w226:cluster{"f0":dbl, "df":dbl, "magnitude":dbl[]})  [unwired: 5 in, 3 out]
        "micfft" <- w226
        n100 = call-poly "fftGetMagsPoly.vi"("input cluster"=w226, "405 F (Hz)"=w225, "532 F (Hz)"=w224, "660 F (Hz)"=w198, "785 F (Hz)"=w203, "unit cal, scu"=w223) -> ("mag405 (mV)"=w218:dbl, "mag532 (mV)"=w217:dbl, "mag660 (mV)"=w216:dbl, "mag785 (mV)"=w199:dbl)  [unwired: 6 in]
        n101 = Bundle("X"=w234, "mag405 (mV)"=w218) -> (w222:cluster{"X":dbl[], "mag405 (mV) ":dbl})  [unwired: 1 in]
        n102 = Bundle("X"=w233, "mag532 (mV)"=w217) -> (w221:cluster{"X":dbl[], "mag532 (mV)":dbl})  [unwired: 1 in]
        n103 = Bundle("X"=w232, "mag660 (mV)"=w216) -> (w220:cluster{"X":dbl[], "mag660 (mV)":dbl})  [unwired: 1 in]
        n104 = Bundle("X"=w200, "mag785 (mV)"=w199) -> (w201:cluster{"X":dbl[], "mag785 (mV)":dbl})  [unwired: 1 in]
        n105 = local read "PAS Save"() -> (w204:bool)
        n106 = local read "mic"() -> (w213:path)
        n107 = call-poly "rollingAverage_multi.vi"("Magnitude Averaging (no. Avgs.)"="rollavg", "785"=w201, "660"=w220, "532"=w221, "405"=w222) -> ("785 Data"=w202:T11, "660 Data"=w209:T12, "532 Data"=w210:T13, "405 Data"=w211:T14)  [unwired: 3 in]
        n108 = call "saveTimeSeries_IV.vi"("1"=w218, "file path (dialog if empty)"=w213, "save?"=w204, "2"=w217, "3"=w216, "4"=w199, "Error In"=w215, "Number of Data Series"=enum16{"1", "2", "3", "4"}."4") -> ("Error Out"=w214:errorcluster)  [unwired: 7 in]
        n109 = call-poly "micUnbundle.vi"("405nm Data"=w211, "532nm Data"=w210, "660nm Data"=w209, "785nm Data"=w202) -> ("pd ts"=w208:T4, "405 New Array"=w207:dbl[], "532 New Array"=w206:dbl[], "660 New Array"=w205:dbl[], "785 New Array"=w197:dbl[])  [unwired: 7 in]
        "mic ts" <- w208
      }
      frame Error {
      }
    }
    n110 = Wait Until Next ms Multiple(millisecond multiple=u32 1000) -> ()  [unwired: 1 out]
    n111 = Enqueue Element(queue=w182, element=w181, error in (no error)=w184) -> (queue out=w183:refnum<queue>, error out=w180:errorcluster)  [unwired: 1 in, 1 out]
  }
  n112 = while {
    shift-right: [w263] -> _
    shift-left: w12 -> [w260]
    shift-right: [w262] -> _
    shift-left: w12 -> [w259]
    shift-right: [w261] -> _
    shift-left: w12 -> [w258]
    tunnel: w29 -> [w256]
    tunnel: w26 -> [w255]
    tunnel: "mic cal, scu" -> [w254]
    shift-right: [w251] -> w18
    shift-left: w15 -> [w252]
    shift-right: [w250] -> w17
    shift-left: w19 -> [w253]
    shift-right: [w243] -> _
    shift-left: w12 -> [w245]
    stop <- w257 stop-if-true
    # "Photodiode Processing Loop (Consumer)"
    n113 = Dequeue Element(queue=w256) -> (element=w264:i32[][], error out=w265:errorcluster)  [unwired: 2 in, 2 out]
    n114 = case shown="Error" w265 {
      selector: w265 -> [_ w311]
      tunnel: w264 -> [w303 _]
      tunnel: w260 -> [w307 w314]
      tunnel: w259 -> [w306 w312]
      tunnel: w258 -> [w305 w313]
      tunnel: [w279 w314] -> w263
      tunnel: [w278 w312] -> w262
      tunnel: [w277 w313] -> w261
      tunnel: [w287 w311] -> w257
      tunnel: w255 -> [w301 _]
      tunnel: w254 -> [w296 _]
      tunnel: "660 PD Cal 3" -> [w274 _]
      tunnel: "532 PD Cal 3" -> [w275 _]
      tunnel: "405 PD Cal 3" -> [w276 _]
      tunnel: [w280 cluster{dbl, dbl, dbl, dbl} {0.0, 0.0, 0.0, 0.0}] -> w249
      tunnel: w245 -> [w272 w309]
      tunnel: "785 PD Cal" -> [w268 _]
      tunnel: [w266 w309] -> w243
      frame No Error {
        w308 = T10 0 items=["Rectangle"=0, "Hanning"=1, "Hamming"=2, "Blackman-Harris"=3, "Exact Blackman"=4, "Blackman"=5, "Flat Top"=6, "4 Term B-Harris "=7, "7 Term B-Harris"=8, "Low Sidelobe"=9, "Blackman Nuttall"=11, "Triangle"=30, "Bartlett-Hanning"=31, "Bohman"=32, "Parzen"=33, "Welch"=34, "Kaiser"=60, "Dolph-Chebyshev"=61, "Gaussian"=62] ("window")
        n115 = Index Array(array=w303, index (row)=0) -> (element=w302:i32[])  [unwired: 1 in]
        n116 = Bundle By Name("Y"=w302, "dt"=w301) -> (w300:waveform(i32))  [unwired: 1 in]
        "pdwave" <- w300
        n117 = local read "423 F (Hz)"() -> (w298:i32)
        n118 = local read "532 F (Hz)"() -> (w297:i32)
        n119 = local read "662 F (Hz)"() -> (w267:i32)
        n120 = local read "785 F (Hz)"() -> (w270:i32)
        n121 = call-poly <vilib>:"FFT Spectrum (Mag-Phase).vi"("window"=w308, "time signal"=w300) -> ("error out"=w288:errorcluster, "magnitude"=w299:cluster{"f0":dbl, "df":dbl, "magnitude":dbl[]})  [unwired: 5 in, 3 out]
        "pdfft" <- w299
        n122 = call-poly "fftGetMagsPoly.vi"("input cluster"=w299, "405 F (Hz)"=w298, "532 F (Hz)"=w297, "660 F (Hz)"=w267, "785 F (Hz)"=w270, "unit cal, scu"=w296) -> ("mag405 (mV)"=w291:dbl, "mag532 (mV)"=w290:dbl, "mag660 (mV)"=w289:dbl, "mag785 (mV)"=w271:dbl)  [unwired: 6 in]
        n123 = Bundle("X"=w307, "mag405 (mV)"=w291) -> (w295:cluster{"X":dbl[], "mag405 (mV) ":dbl})  [unwired: 1 in]
        n124 = Bundle("X"=w306, "mag532 (mV)"=w290) -> (w294:cluster{"X":dbl[], "mag532 (mV)":dbl})  [unwired: 1 in]
        n125 = Bundle("X"=w305, "mag660 (mV)"=w289) -> (w293:cluster{"X":dbl[], "mag660 (mV)":dbl})  [unwired: 1 in]
        n126 = Bundle("X"=w272, "mag785 (mV)"=w271) -> (w273:cluster{"X":dbl[], "mag785 (mV)":dbl})  [unwired: 1 in]
        n127 = local read "PAS Save"() -> (w286:bool)
        n128 = local read "pd"() -> (w285:path)
        n129 = call-poly "rollingAverage_multi.vi"("Magnitude Averaging (no. Avgs.)"="Chart Rolling Average", "785"=w273, "660"=w293, "532"=w294, "405"=w295) -> ("785 Data"=w269:T11, "660 Data"=w281:T12, "532 Data"=w282:T13, "405 Data"=w283:T14)  [unwired: 3 in]
        n130 = call "saveTimeSeries_IV.vi"("1"=w291, "file path (dialog if empty)"=w285, "save?"=w286, "2"=w290, "3"=w289, "Error In"=w288, "Number of Data Series"=enum16{"1", "2", "3", "4"}."4") -> ("Error Out"=w287:errorcluster)  [unwired: 8 in]
        n131 = call-poly "pdNormalize.vi"("405 Data"=w283, "532 Data"=w282, "660 Data"=w281, "785 Data"=w269, "785 PD Cal"=w268, "405 PD Cal"=w276, "532 PD Cal"=w275, "660 PD Cal"=w274) -> ("Output Cluster"=w280:cluster{dbl, dbl, dbl, dbl}, "405 New Array"=w279:dbl[], "532 New Array"=w278:dbl[], "660 New Array"=w277:dbl[], "785 New Array"=w266:dbl[])  [unwired: 3 in]
        "pd ts" <- w280
      }
      frame Error {
      }
    }
    n132 = Wait Until Next ms Multiple(millisecond multiple=u32 1000) -> ()  [unwired: 1 out]
    n133 = Enqueue Element(queue=w252, element=w249, error in (no error)=w253) -> (queue out=w251:refnum<queue>, error out=w250:errorcluster)  [unwired: 1 in, 1 out]
  }
  n134 = while {
    tunnel: w16 -> [w317]
    tunnel: w15 -> [w316]
    stop <- w322 stop-if-true
    # "This loop takes data from the two FFT loops and converts to absorption via the calibration."
    # "Absorption Data Loop (Consummer II)"
    n135 = Dequeue Element(queue=w317) -> (element=w323:cluster{dbl, dbl, dbl, dbl}, error out=w321:errorcluster)  [unwired: 2 in, 2 out]
    n136 = Dequeue Element(queue=w316) -> (element=w318:cluster{dbl, dbl, dbl, dbl}, error out=w320:errorcluster)  [unwired: 2 in, 2 out]
    n137 = Wait Until Next ms Multiple(millisecond multiple=u32 1000) -> ()  [unwired: 1 out]
    n138 = Merge Errors(w321, w320) -> (w319:errorcluster)
    n139 = case shown="No Error" w319 {
      selector: w319 -> [w331 w333]
      tunnel: w323 -> [_ _]
      tunnel: [w330 w333] -> w322
      tunnel: w318 -> [_ _]
      frame No Error {
        n140 = local read "processed"() -> (w327:path)
        n141 = local read "PAS Save"() -> (w328:bool)
        n142 = call-poly "absCalcPlot.vi"("file path (dialog if empty)"=w327, "Cell Calibration, mV/mW"="cellcal", "save?"=w328, "Error In"=w331, "bkg values"="Bkg Values (mV)") -> ("Error Out"=w330:errorcluster, "aae"=→"AAE":dbl, "b_abs/ext ts"=→"abs/ext":cluster{dbl, dbl, dbl, dbl, "crd":dbl}, "Spectrum"=→"Absorption Spectrum":cluster{dbl[], "Best Power Fit":dbl[]}[])  [unwired: 3 in]
      }
      frame Error {
      }
    }
  }
  n143 = while "Message Processor" {
    shift-left: w74 -> [w347]
    shift-right: [w339] -> w70
    tunnel: w60 -> [w346]
    shift-left: "State Variables" -> [w352]
    shift-right: [w351] -> _
    tunnel: "406 Port" -> [w343]
    tunnel: "532 Port" -> [w342]
    tunnel: "662 Port" -> [w341]
    tunnel: "Teensy Port" -> [w340]
    shift-right: [w337] -> _
    shift-left: _ -> [w336]
    tunnel: "785 Port" -> [w334]
    stop <- w350 stop-if-true
    w344 = 100  # Timeout
    n144 = call "QMH Get Next Message from Queue.vi"("error in (no error)"=w347, "ms timeout (1)"=w344, "queue in"=w346) -> ("error out"=w348:errorcluster, "Next Parameter"=w335:string, "Next Message"=w345:string, "queue out"=w349:refnum<queue>, "Stop QMH"=w350:bool)  [unwired: 3 in]
    n145 = case shown="\"filter\"" w345 {
      selector: w345 -> [_ w380 _ _ _ _ _ _ _ _ _ _ _ _ _ _ _ _ _ _ _ _]
      tunnel: [w376 w381 w396 w407 w470 w501 w503 w510 w516 w522 w528 w534 w542 w549 w556 w563 w584 w591 w616 w627 w640 w652] -> w351
      tunnel: w352 -> [w376 w381 w396 w407 w470 w501 w503 w510 w516 w522 w528 w534 w542 w549 w556 w563 w584 w591 w616 w627 w640 w652]
      tunnel: w349 -> [_ _ _ w400 _ _ _ _ _ _ _ _ _ _ _ _ _ _ _ _ w638 w653]
      tunnel: w348 -> [w368 w377 w394 w406 w468 w500 w506 w512 w518 w524 w527 w530 w539 w546 w554 w561 w585 w588 w614 w626 w639 w654]
      tunnel: [w364 w377 w387 w399 w467 w496 w502 w508 w514 w521 w527 w533 w540 w547 w555 w557 w585 w587 w613 w626 w636 w643] -> w339
      tunnel: w343 -> [w370 _ w395 w398 _ _ w505 _ _ _ _ w535 _ _ _ w560 _ _ _ _ _ w649]
      tunnel: w342 -> [w369 _ w392 w402 _ _ _ w509 _ _ _ _ w541 _ _ w559 _ _ _ _ _ w648]
      tunnel: w341 -> [w363 _ w391 w405 _ _ _ _ w515 _ _ _ _ w548 _ w558 _ _ _ _ _ w647]
      tunnel: w340 -> [_ _ w389 w401 w469 w495 _ _ _ _ _ _ _ _ _ _ _ w589 w615 _ _ w650]
      tunnel: w335 -> [_ _ _ _ w466 w499 _ _ _ _ _ w532 w536 w543 w551 _ _ _ w612 w625 _ _]
      tunnel: w334 -> [w367 _ w382 w397 _ _ _ _ _ w520 _ _ _ _ w550 _ _ _ _ _ _ w641]
      frame "", "Wait" {
        # "Update the front panel"
        # "Idle Case - this case is called after a Timeout on the Get Next Message from Queue VI, if no new messages are present on the queue. This case can be used for housekeeping tasks such as updating the UI."
        n146 = Get Date/Time String(want seconds? (F)=TRUE) -> (date string=w375:string, time string=w374:string)  [unwired: 2 in]
        n147 = call-poly "laserDiagnose.vi"("405 Port"=w370, "532 Port"=w369, "660 Port"=w363, "785 Port"=w367, "error in (no error)"=w368) -> ("Temperatures"=→"Laser Temperatures":T3, "Overtemp"=→"Overtemp":bool, "error out"=w364:errorcluster)  [unwired: 6 in, 2 out]
        n148 = Concatenate Strings(w375, " " ("string"), w374) -> (→"Status":string)
      }
      frame Default {
        # "Call this case if a message is received that is not handled \nby any other case. Typically this is a programming error\nas a result of a typo or unhandled message/missing message handler."
        n149 = Format Into String(format string="DevError: Missing message handler for '%s\" message." ("message"), w380) -> (resulting string=w378:string)  [unwired: 2 in, 1 out]
        n150 = One Button Dialog(message=w378) -> ()  [unwired: 1 in, 1 out]
      }
      frame "Initialize" {
        w383 = u32 115200 ("baud rate (9600)")
        # "Initialize the state variables and user interface\nInitialize serial connections"
        n151 = call-poly "VISA Configure Serial Port"("VISA resource name"=w395, "baud rate (9600)"=w383, "error in (no error)"=w394) -> ("error out"=w393:errorcluster)  [unwired: 11 in, 1 out]
        n152 = call-poly "VISA Configure Serial Port"("VISA resource name"=w392, "baud rate (9600)"=w383, "error in (no error)"=w393) -> ("error out"=w390:errorcluster)  [unwired: 11 in, 1 out]
        n153 = call-poly "VISA Configure Serial Port"("VISA resource name"=w391, "baud rate (9600)"=w383, "error in (no error)"=w390) -> ("error out"=w385:errorcluster)  [unwired: 11 in, 1 out]
        n154 = call-poly "VISA Configure Serial Port"("VISA resource name"=w382, "baud rate (9600)"=w383, "error in (no error)"=w385) -> ("error out"=w384:errorcluster)  [unwired: 11 in, 1 out]
        n155 = call-poly "VISA Configure Serial Port"("VISA resource name"=w389, "error in (no error)"=w384) -> ("VISA resource name out"=w388:refnum<visa-resource-name>, "error out"=w386:errorcluster)  [unwired: 12 in]
        n156 = property class="Instr" props=["Baud"](reference=w388, error in=w386) -> (error out=w387:errorcluster)  [unwired: 2 out]
      }
      frame "sweep" {
        # "Perform a frequency sweep and calculate the resonance frequency"
        n157 = stacked-sequence {
          seq-local: [_ w422 _ _] -> [_ _ w450 _]
          tunnel: w406 -> [_ w416 _ _]
          tunnel: "Data End Frequency (Hz)" -> [_ w419 w444 _]
          tunnel: "Data Start Frequency (Hz)" -> [_ w418 w443 _]
          tunnel: w405 -> [w413 _ _ w460]
          tunnel: w402 -> [w411 _ _ w459]
          tunnel: w401 -> [_ w417 _ _]
          tunnel: w400 -> [_ _ _ w464]
          tunnel: [_ _ _ w461] -> w399
          tunnel: w398 -> [_ _ _ _]
          tunnel: w397 -> [w408 _ _ w455]
          frame #0 {
            w409 = FALSE
            # "Turn red, green, IR lasers off for scan."
            n158 = call "laserOnOff.vi"("Emission (F = OFF)"=w409, "VISA Refnum in"=w411) -> ("error out"=w415:errorcluster)  [unwired: 7 in, 2 out]
            n159 = Wait (ms)(milliseconds to wait=u32 5000) -> ()  [unwired: 1 out]
            n160 = local write "Status"("Conducting Frequency Sweep" ("Status")) -> ()
            n161 = call "laserOnOff.vi"("error in (no error)"=w415, "Emission (F = OFF)"=w409, "VISA Refnum in"=w413) -> ("error out"=w410:errorcluster)  [unwired: 6 in, 2 out]
            n162 = call "laserOnOff.vi"("error in (no error)"=w410, "Emission (F = OFF)"=w409, "VISA Refnum in"=w408) -> ()  [unwired: 6 in, 3 out]
          }
          frame #1 {
            n163 = Subtract(x=w419, y=w418) -> (x-y=w420:i32)
            n164 = for {
              N: w420 -> [w426]
              tunnel: [w431] -> w422 mode=indexing
              tunnel: w418 -> [w430]
              tunnel: w419 -> [w429]
              tunnel: w416 -> [_]
              i -> [w423]
              # "Get microphone data."
              # "Listen for N*2000\n seconds"
              n165 = Increment(x=w423) -> (x+1=w424:i32)
              n166 = Divide(x=w424, y=w426) -> (x/y=→"sweep progress":dbl)
              n167 = local read "micfft"() -> (w428:cluster{"f0":dbl, "df":dbl, "magnitude":dbl[]})
              n168 = Unbundle By Name(w428) -> ("magnitude"=w427:dbl[])
              n169 = Wait (ms)(milliseconds to wait=u32 2000) -> ()  [unwired: 1 out]
              n170 = call "fftGetMax.vi"("End Frequency (Hz)"=w429, "Start Frequency (Hz)"=w430, "Magnitudes"=w427) -> ("max value"=w431:dbl)  [unwired: 8 in]
            }
            n171 = case shown="False" TRUE ("sweep?") {
              tunnel: w418 -> [_ w438]
              tunnel: w419 -> [_ w437]
              tunnel: w417 -> [_ w436]
              tunnel: [w433 w435] -> _
              tunnel: w416 -> [w433 w434]
              frame False {
              }
              frame True {
                # "Scan laser freq.\nwith Teensy"
                n172 = call "teensySweepFreq.vi"("error in (no error)"=w434, "end f, Hz (1385)"=w437, "start f, Hz (1355)"=w438, "VISA Refnum in"=w436) -> ("error out"=w435:errorcluster)  [unwired: 7 in]
              }
            }
          }
          frame #2 {
            # "Calculate resonance frequency;\ndisplay and save scan."
            n173 = Wait (ms)(milliseconds to wait=u32 5000) -> ()  [unwired: 1 out]
            n174 = local read "PAS Save"() -> (w439:bool)
            n175 = To Double Precision Float(number=w444) -> (double precision float=w441:dbl)
            n176 = To Double Precision Float(number=w443) -> (double precision float=w442:dbl)
            n177 = call "resCalc.vi"("Frequency Sweep"=w450, "Start F, Hz (1355)"=w443) -> ("F-res, Hz"=w448:dbl, "Frequency Scan"=w440:cluster{i32[], "Best Gaussian Fit":dbl[]}[])  [unwired: 8 in]
            "freqscan" <- w440
            n178 = In Range and Coerce(upper limit=w441, x=w448, lower limit=w442) -> (In Range?=w447:bool)  [unwired: 1 out]
            n179 = case shown="True" w439 {
              tunnel: w440 -> [_ w454]
              tunnel: w448 -> [_ w453]
              frame False {
              }
              frame True {
                n180 = local read "sweeps"() -> (w452:path)
                n181 = call "saveFreqSweep.vi"("f-res, Hz"=w453, "Frequency Scan"=w454, "file path (dialog if empty)"=w452) -> ()  [unwired: 9 in]
              }
            }
            n182 = And(x=w447, y=TRUE ("check freqs?")) -> (x .and. y?=w445:bool)
            n183 = case shown="True" w445 {
              tunnel: w448 -> [_ w451]
              frame False {
              }
              frame True {
                n184 = property on="Calculated Resonance (Hz)" class="DigNum (strict)"("Val(Sgnl)"=w451) -> ()  [unwired: 2 in, 2 out]
                "Calculated Resonance (Hz)" <- w451
              }
            }
          }
          frame #3 {
            w456 = TRUE
            # "Turn red, green, IR lasers back on."
            n185 = call "laserOnOff.vi"("Emission (F = OFF)"=w456, "VISA Refnum in"=w459) -> ("error out"=w465:errorcluster)  [unwired: 7 in, 2 out]
            n186 = call "laserOnOff.vi"("error in (no error)"=w465, "Emission (F = OFF)"=w456, "VISA Refnum in"=w460) -> ("error out"=w458:errorcluster)  [unwired: 6 in, 2 out]
            n187 = call "laserOnOff.vi"("error in (no error)"=w458, "Emission (F = OFF)"=w456, "VISA Refnum in"=w455) -> ("error out"=w457:errorcluster)  [unwired: 6 in, 2 out]
            n188 = call-poly "QMH Add Message to Queue.vi"("error in (no error)"=w457, "Parameter"="532 F (Hz)", "Message"="freqset", "queue in"=w464) -> ("error out"=w461:errorcluster)  [unwired: 6 in, 1 out]
          }
        }
      }
      frame "freqset" {
        # "Set the frequency of the Teensy's modulation\nsignal for single laser (if single frequency is changed)."
        # "Set the laser frequency.  Case for \"red\", \"blue\", or \"green\"."
        n189 = case shown="\"405 F (Hz) \", Default" w466 {
          tunnel: w468 -> [w475 w480 w484 w490]
          tunnel: [w474 w479 w483 w489] -> w467
          tunnel: w469 -> [w471 w476 w481 w488]
          frame "405 F (Hz) ", Default {
            w473 = u16 0 items=["blue", "green", "red"] ("laser")
            n190 = call "freqSet.vi"("error in (no error)"=w475, "laser"=w473, "Freq, Hz (1370)"="423 F (Hz)", "Teensy Port"=w471) -> ("error out"=w474:errorcluster)  [unwired: 6 in, 1 out]
          }
          frame "532 F (Hz)" {
            w478 = u16 1 items=["blue", "green", "red"] ("laser")
            n191 = call "freqSet.vi"("error in (no error)"=w480, "laser"=w478, "Freq, Hz (1370)"="532 F (Hz)", "Teensy Port"=w476) -> ("error out"=w479:errorcluster)  [unwired: 6 in, 1 out]
          }
          frame "662 F (Hz)" {
            w485 = u16 2 items=["blue", "green", "red"] ("laser")
            n192 = call "freqSet.vi"("error in (no error)"=w484, "laser"=w485, "Freq, Hz (1370)"="662 F (Hz)", "Teensy Port"=w481) -> ("error out"=w483:errorcluster)  [unwired: 6 in, 1 out]
          }
          frame "785 F (Hz)" {
            w486 = u16 3 items=["blue", "green", "red", "ir"] ("laser")
            n193 = call "freqSet.vi"("error in (no error)"=w490, "laser"=w486, "Freq, Hz (1370)"="785 F (Hz)", "Teensy Port"=w488) -> ("error out"=w489:errorcluster)  [unwired: 6 in, 1 out]
          }
        }
      }
      frame "setfreqs" {
        # "Set the frequency of the Teensy's modulation\nsignal for all lasers at once."
        # "Set laser frequencies to resonance frequency calculated in sweep."
        n194 = Scan From String(input string=w499, error in=w500) -> (error out=w497:errorcluster, output 1=w498:dbl)  [unwired: 3 in, 2 out]
        n195 = call-poly "lasersSetFrequencies.vi"("VISA Refnum in"=w495, "f-res (Hz)"=w498, "error in (no error)"=w497) -> ("405 f (Hz)"=w494:i32, "532 f (Hz)"=w493:i32, "662 f (Hz)"=w492:i32, "785 f (Hz)"=w491:i32, "error out"=w496:errorcluster)  [unwired: 8 in]
        n196 = local write "662 F (Hz)"(w492) -> ()
        n197 = local write "532 F (Hz)"(w493) -> ()
        n198 = local write "423 F (Hz)"(w494) -> ()
        n199 = local write "785 F (Hz)"(w491) -> ()
      }
      frame "405 emit" {
        # "Turn laser on or off"
        n200 = call "laserOnOff.vi"("error in (no error)"=w506, "Emission (F = OFF)"="406 Emission", "Power, mW (100)"="406 Power (mW)", "VISA Refnum in"=w505) -> ("error out"=w502:errorcluster)  [unwired: 5 in, 2 out]
      }
      frame "532 emit" {
        # "Turn laser on or off"
        n201 = call "laserOnOff.vi"("error in (no error)"=w512, "Emission (F = OFF)"="532 Emission", "Power, mW (100)"="532 Power (mW)", "VISA Refnum in"=w509) -> ("error out"=w508:errorcluster)  [unwired: 5 in, 2 out]
      }
      frame "660 emit" {
        # "Turn laser on or off"
        n202 = call "laserOnOff.vi"("error in (no error)"=w518, "Emission (F = OFF)"="662 Emission", "Power, mW (100)"="662 Power (mW)", "VISA Refnum in"=w515) -> ("error out"=w514:errorcluster)  [unwired: 5 in, 2 out]
      }
      frame "785 emit" {
        # "Turn laser on or off"
        n203 = call "laserOnOff.vi"("error in (no error)"=w524, "Emission (F = OFF)"="785 Emission", "Power, mW (100)"="785 Power (mW)", "VISA Refnum in"=w520) -> ("error out"=w521:errorcluster)  [unwired: 5 in, 2 out]
      }
      frame "emit" {
        # "Turn on all lasers."
        n204 = local write "406 Emission"("All Emit") -> ()
        n205 = local write "532 Emission"("All Emit") -> ()
        n206 = local write "662 Emission"("All Emit") -> ()
        n207 = local write "785 Emission"("All Emit") -> ()
      }
      frame "405 Power" {
        # "Set laser power"
        n208 = Scan From String(input string=w532, error in=w530) -> (error out=w529:errorcluster, output 1=w531:dbl)  [unwired: 3 in, 2 out]
        n209 = call "laserSetPower.vi"("error in (no error)"=w529, "Laser Power (mW)"=w531, "VISA Refnum in"=w535) -> ("error out"=w533:errorcluster)  [unwired: 7 in, 1 out]
      }
      frame "532 Power" {
        n210 = Scan From String(input string=w536, error in=w539) -> (error out=w538:errorcluster, output 1=w537:dbl)  [unwired: 3 in, 2 out]
        n211 = call "laserSetPower.vi"("error in (no error)"=w538, "Laser Power (mW)"=w537, "VISA Refnum in"=w541) -> ("error out"=w540:errorcluster)  [unwired: 7 in, 1 out]
      }
      frame "660 Power" {
        n212 = Scan From String(input string=w543, error in=w546) -> (error out=w545:errorcluster, output 1=w544:dbl)  [unwired: 3 in, 2 out]
        n213 = call "laserSetPower.vi"("error in (no error)"=w545, "Laser Power (mW)"=w544, "VISA Refnum in"=w548) -> ("error out"=w547:errorcluster)  [unwired: 7 in, 1 out]
      }
      frame "785 Power" {
        n214 = Scan From String(input string=w551, error in=w554) -> (error out=w553:errorcluster, output 1=w552:dbl)  [unwired: 3 in, 2 out]
        n215 = call "laserSetPower.vi"("error in (no error)"=w553, "Laser Power (mW)"=w552, "VISA Refnum in"=w550) -> ("error out"=w555:errorcluster)  [unwired: 7 in, 1 out]
      }
      frame "align" {
        # "Set power of all lasers to 5 mW for alignment"
        n216 = case shown="True" "Alignment Mode" {
          tunnel: w561 -> [w571 w581]
          tunnel: w560 -> [w570 w580]
          tunnel: w559 -> [w569 w579]
          tunnel: w558 -> [w568 w578]
          tunnel: [w565 w575] -> w557
          frame True {
            w564 = 5.0 ("Laser Power (mW)")
            n217 = call "laserSetPower.vi"("error in (no error)"=w571, "Laser Power (mW)"=w564, "VISA Refnum in"=w570) -> ("error out"=w567:errorcluster)  [unwired: 7 in, 1 out]
            n218 = call "laserSetPower.vi"("error in (no error)"=w567, "Laser Power (mW)"=w564, "VISA Refnum in"=w569) -> ("error out"=w566:errorcluster)  [unwired: 7 in, 1 out]
            n219 = call "laserSetPower.vi"("error in (no error)"=w566, "Laser Power (mW)"=w564, "VISA Refnum in"=w568) -> ("error out"=w565:errorcluster)  [unwired: 7 in, 1 out]
          }
          frame False, Default {
            n220 = local read "406 Power (mW)"() -> (w574:dbl)
            n221 = local read "532 Power (mW)"() -> (w573:dbl)
            n222 = local read "662 Power (mW)"() -> (w572:dbl)
            n223 = call "laserSetPower.vi"("error in (no error)"=w581, "Laser Power (mW)"=w574, "VISA Refnum in"=w580) -> ("error out"=w577:errorcluster)  [unwired: 7 in, 1 out]
            n224 = call "laserSetPower.vi"("error in (no error)"=w577, "Laser Power (mW)"=w573, "VISA Refnum in"=w579) -> ("error out"=w576:errorcluster)  [unwired: 7 in, 1 out]
            n225 = call "laserSetPower.vi"("error in (no error)"=w576, "Laser Power (mW)"=w572, "VISA Refnum in"=w578) -> ("error out"=w575:errorcluster)  [unwired: 7 in, 1 out]
          }
        }
      }
      frame "background" {
        n226 = local read "mic ts"() -> (w583:T4)
        n227 = local read "Tau_662 vs. T"() -> (w582:dbl)
        n228 = local write "Bkg Values (mV)"(w583) -> ()
        n229 = local write "tau_0 (us)"(w582) -> ()
      }
      frame "filter" {
        n230 = local read "Filtering"() -> (w590:bool)
        n231 = case shown="True" w590 {
          tunnel: w589 -> [w594 w603]
          tunnel: w588 -> [w593 w601]
          tunnel: [w592 w602] -> w587
          frame False {
            n232 = Multiply(x="Filter Length (min)", y=60.0) -> (x*y=w597:dbl)
            n233 = local write "Time Target (s)"(w597) -> ()
            n234 = VISA Write(VISA resource name=w594, write buffer="v.1", error in (no error)=w593) -> (error out=w592:errorcluster)  [unwired: 2 out]
            "Filtering" <- TRUE
          }
          frame True {
            n235 = flat-sequence {
              tunnel: w601 -> [w611]
              tunnel: [w611] -> w600
              frame #0 {
                n236 = local read "Tau_662 vs. T"() -> (w609:dbl)
                n237 = local read "mic ts"() -> (w610:T4)
                n238 = local write "Bkg Values (mV)"(w610) -> ()
                n239 = local write "tau_0 (us)"(w609) -> ()
              }
            }
            n240 = local write "Filtering"(FALSE) -> ()
            n241 = VISA Write(VISA resource name=w603, write buffer="v.0", error in (no error)=w600) -> (error out=w602:errorcluster)  [unwired: 2 out]
            n242 = Multiply(x="Sample Length (min)", y=60.0) -> (x*y=w605:dbl)
            n243 = local write "Time Target (s)"(w605) -> ()
          }
        }
        n244 = Wait (ms)(milliseconds to wait=u32 500) -> ()  [unwired: 1 out]
      }
      frame "filterswitch" {
        n245 = case shown="\"TRUE\"" w612 {
          tunnel: w615 -> [w619 w624]
          tunnel: w614 -> [w618 w623]
          tunnel: [w617 w622] -> w613
          frame "FALSE", Default {
            n246 = VISA Write(VISA resource name=w619, write buffer="v.0", error in (no error)=w618) -> (error out=w617:errorcluster)  [unwired: 2 out]
          }
          frame "TRUE" {
            n247 = VISA Write(VISA resource name=w624, write buffer="v.1", error in (no error)=w623) -> (error out=w622:errorcluster)  [unwired: 2 out]
          }
        }
      }
      frame "namefiles" {
        n248 = case shown="\"TRUE\"" w625 {
          frame "FALSE", Default {
            n249 = local write "PAS Save"(FALSE ("PAS Save")) -> ()
          }
          frame "TRUE" {
            n250 = flat-sequence {
              frame #0 {
                n251 = call "saveSetDirectory.vi"() -> ("mic"=→"mic":path, "pd"=→"pd":path, "processed"=→"processed":path, "sweeps"=→"sweeps":path, "crd"=→"crd":path)  [unwired: 11 in]
              }
              frame #1 {
                "PAS Save" <- TRUE ("PAS Save")
              }
            }
          }
        }
      }
      frame "Error" {
        (unwired) errorcluster {"status"=FALSE, "code"=0, "source"=""} ("error out")
        # "Proceed to Exit - remove if this is\nnot appropriate for the General Error case"
        # "General Error Case - this case is called if an error is passed using the error cluster below. Typically most new errors should be handed in each individual case and not passed in the rror cluster. If necessary a custom error handler case should be added and called from other cases."
        n252 = call <vilib>:"Simple Error Handler.vi"("error in (no error)"=w639) -> ("error out"=w635:errorcluster)  [unwired: 4 in, 4 out]
        n253 = call-poly "QMH Add Message to Queue.vi"("error in (no error)"=w635, "Message"="Exit", "queue in"=w638) -> ("error out"=w636:errorcluster)  [unwired: 7 in, 1 out]
      }
      frame "Exit" {
        # "Perform cleanup tasks: Close serial connections and clear front panel."
        n254 = call "QMH Destroy Queue.vi"("error in (no error)"=w654, "queue in"=w653) -> ("error out"=w646:errorcluster)  [unwired: 7 in, 2 out]
        n255 = for {
          N: 4 -> [_]
          tunnel: w649 -> [w662]
          tunnel: w648 -> [w660]
          tunnel: w647 -> [w659]
          tunnel: w646 -> [w658]
          tunnel: FALSE -> [w657]
          tunnel: [w656] -> w642
          tunnel: w641 -> [w655]
          i -> [w661]
          # "Close laser serial connections."
          n256 = case shown="0, Default" w661 {
            tunnel: [w669 w674 w679 w684] -> w664
            tunnel: [w668 w673 w678 w683] -> w663
            tunnel: w662 -> [w667 _ _ _]
            tunnel: w660 -> [_ w672 _ _]
            tunnel: w659 -> [_ _ w676 _]
            tunnel: w658 -> [w666 w671 w677 w682]
            tunnel: w657 -> [w665 w670 w675 w681]
            tunnel: w655 -> [_ _ _ w680]
            frame 0, Default {
              n257 = call "laserOnOff.vi"("error in (no error)"=w666, "Emission (F = OFF)"=w665, "VISA Refnum in"=w667) -> ("error out"=w669:errorcluster, "VISA Refnum out"=w668:refnum<visa-resource-name>)  [unwired: 6 in, 1 out]
              n258 = local write "406 Emission"(w665) -> ()
            }
            frame 1 {
              n259 = call "laserOnOff.vi"("error in (no error)"=w671, "Emission (F = OFF)"=w670, "VISA Refnum in"=w672) -> ("error out"=w674:errorcluster, "VISA Refnum out"=w673:refnum<visa-resource-name>)  [unwired: 6 in, 1 out]
              n260 = local write "532 Emission"(w670) -> ()
            }
            frame 2 {
              n261 = call "laserOnOff.vi"("error in (no error)"=w677, "Emission (F = OFF)"=w675, "VISA Refnum in"=w676) -> ("error out"=w679:errorcluster, "VISA Refnum out"=w678:refnum<visa-resource-name>)  [unwired: 6 in, 1 out]
              n262 = local write "662 Emission"(w675) -> ()
            }
            frame 3 {
              n263 = call "laserOnOff.vi"("error in (no error)"=w682, "Emission (F = OFF)"=w681, "VISA Refnum in"=w680) -> ("error out"=w684:errorcluster, "VISA Refnum out"=w683:refnum<visa-resource-name>)  [unwired: 6 in, 1 out]
              n264 = local write "785 Emission"(w681) -> ()
              n265 = local write "All Emit"(w681) -> ()
            }
          }
          n266 = VISA Close(VISA resource name=w663, error in (no error)=w664) -> (error out=w656:errorcluster)
        }
        n267 = local write "Status"("" ("Status")) -> ()
        n268 = VISA Close(VISA resource name=w650, error in (no error)=w642) -> (error out=w643:errorcluster)
      }
    }
    n269 = case shown="True" "Auto Filter" {
      tunnel: [w353 w355] -> w337
      tunnel: w336 -> [w353 w354]
      frame False {
      }
      frame True {
        # "This is the timer for the filtering routine."
        n270 = call "Elapsed Time"("Time Target (s)"="Time Target (s)", "Auto Reset"=TRUE, "error in (no error)"=w354) -> ("Elapsed Time (s)"=w358:dbl, "Time has Elapsed"=w360:bool, "error out"=w359:errorcluster)  [unwired: 9 in, 5 out]
        "Time has Elapsed" <- w360
        n271 = Divide(x=w358, y=60.0) -> (x/y=→"Elapsed Time (min)":dbl)
        n272 = property on="Time has Elapsed" class="Bool (strict)"(error in=w359, "Val(Sgnl)"=w360) -> (error out=w355:errorcluster)  [unwired: 1 in, 1 out]
      }
    }
  }
  n273 = while {
    shift-right: [w696] -> _
    shift-left: w2 -> [w697]
    stop <- w693 stop-if-true
    # "CRD Consumer: Fit & Calculate RDT"
    n274 = case shown="True" "fast" {
      frame False {
      }
      frame True {
        n275 = Wait Until Next ms Multiple(millisecond multiple=u32 1000) -> ()  [unwired: 1 out]
      }
    }
    n276 = call "crd_processWaveform.vi"("No Avg."="No. Averages", "Queue in"=w697) -> ("error out"=w694:errorcluster, "tau (us)"=w689:dbl, "Decay"=→"Decay":cluster{sgl[], "Best Exponential Fit":dbl[]}[], "Queue out"=w696:refnum<queue>)  [unwired: 6 in]
    "Tau_662 vs. T" <- w689
    n277 = call "crdCalcExtinction.vi"("R_l"=1.18, "tau_0 (us)"="tau_0 (us)", "tau (us)"=w689) -> ("b_ext (1/Mm)"=w686:dbl)  [unwired: 8 in]
    "b_ext (1/Mm)" <- w686
    n278 = local read "PAS Save"() -> (w690:bool)
    n279 = local read "crd"() -> (w691:path)
    n280 = call-poly "saveTimeSeries.vi"("1"=w689, "file path (dialog if empty)"=w691, "save?"=w690, "2"=w686, "Error In"=w694, "Number of Data Series"=enum16{"1", "2", "3", "4"}."2") -> ("Error Out"=w693:errorcluster)  [unwired: 9 in]
  }
  n281 = call "PicoScope2000aClose.vi"("handle"=w1) -> ()
  n282 = Release Queue(queue=w4, error in (no error)=w3) -> ()  [unwired: 1 in, 3 out]
  n283 = Release Queue(queue=w21, error in (no error)=w20) -> ()  [unwired: 1 in, 3 out]
  n284 = Merge Errors(w70, w61) -> (w69:errorcluster)
  n285 = Release Queue(queue=w18, error in (no error)=w17) -> ()  [unwired: 1 in, 3 out]
  n286 = call <vilib>:"Simple Error Handler.vi"("error in (no error)"=w69) -> ("error out"=w68:errorcluster)  [unwired: 4 in, 4 out]
  n287 = flat-sequence {
    tunnel: w68 -> [w700]
    tunnel: [w700] -> w67
    frame #0 {
      n288 = local write "Exit"(FALSE) -> ()
    }
  }
  "Error Console" <- w67
